vi "Argos_K_0v7.vi"(0 "PID 1 COM":refnum<visa-resource-name>="COM1", 1 "Setpoint\n START":bool, 2 "Write to File":bool, 3 "SP 1 input (°C)":dbl=20.0 min=0.0 max=1300.0, 4 "Intervall (s)":u32=1 max=600, 5 "Write/\nRead":bool=TRUE, 6 "Delay (ms)":u32=500 min=100 max=600000, 7 "Auto Tune":bool, 9 "Standby":bool, 11 "Reset\nSTOPP":bool, 12 "ON":bool=TRUE caption="OFF", 13 "Get Values":bool, 15 "File Path":path) -> (8 "(°C)":dbl format="%#.3f", 14 "SP 1 is (°C)":dbl)   [LabVIEW 2013]
doc: "1. Verwendung\n\nDas Programm dient der Steuerung und Abfrage des Thermocontrollers I3252 und dem Auslesen von zwei VC 840 Messgeräten und einem Druckmessgerät Pfeiffer Single Gauge. \nDie Messgeräte werden Standardmäßig ausgelesen und erst nach Betätigung des Schalters \"Write to File\" in einer Textdatei abgespeichert. Das Eingabefeld \"Intervall\" legt den Abstand der Messpunkte fest.\nDer Setpoint für den Thermocontroller wird erst nach Betätigung des Tasters \"Setpoint START\" übernommen und angesteuert. Er wird ind den EEPROM des Gerätes geschrieben. Die Regelung kann mit Hilfe des Schalters \"Standby\" unterbrochen werden. Durch den Taster \"Reset STOPP\" kann der Setpoint aus dem EEPROM gelöscht werden.\nDie Eingabeflächen \"Constant\" und \"Thickness\" dienen der Berechnung des spezifischen Widerstands.\nDie Eingabeflächen \"User\" und \"Sample\" werden in den Header der Textdatei übernommen.\nDer Indikator \"File Path\" zeigt den aktuellen Speicherort der Textdatei an. Dieser wird nach ausschalten des Schalters \"Write to File\" gelöscht. Bei erneuten Schreiben muss ein neuer Speicherort gewählt werden. Bei Wahl desselben Speicherorts werden sämtliche bereits gespeicherte Daten gelöscht.\n\n\n2. Erläuterungen zum Blockdiagramm\n2.1 äußere Sequenz\nDie äußerte Sequenz besteht aus fünf Frames. Der erste dient der Initialisierung der Ports. Der zweite dient als Verzögerung um dem Programm genug Zeit zu geben die Ports zu öffnen. Jedoch senden die beiden VC 840 bereits Informationen an den Computer die in einem Puffer zwischengespeichert werden. Im dritten Frame wird dieser Puffer geleert. Somit kommt es zu keinem Framing Error. Desweiteren wird in diesem Frame die Startzeit der Messungen genommen. Im vierten Frame wird die eigentliche Messung und Verarbeitung der Daten durchgeführt. Die while-Schleife wird nur durch Auftreten eines Fehlers oder durch Betätigung des Stopbuttons auf dem Front Panel in der oberen linken Ecke unterbrochen. Im fünften und letzten Frame werden die Ports wieder geschlossen und beim Auftreten eines Fehlers wird das Programm automatisch gestoppt. Falls kein Fehler auftritt wird die Sequenz von vorne abgearbeitet.\n\n2.2 while-Schleife und innere Sequenz\n2.2.1 \"Event Structure\"\n2.2.1.1 Allgemein\nDer erste Frame beinhaltet ein \"Event Structure\". Dieser reagiert auf insgesamt elf verschiedene Ereignisse. Falls keines dieser Ereignisse auftreten sollte, warte die Struktur eine Millisekunde bevor die \"Event Structure\" verlassen wird. Die übrigen Ereignisse treten ein, wenn der entsprechende Kontroller eine Werteänderung erfährt.\n\n2.2.1.2 Event: Setpoint\nDieser Case besteht von außen nach innen aus einer Stacked Sequence, einer for-Loop und einer Flat Sequence die wiederum zwei \"Case Structures\" enthält. Als erstes wird bei dem Schalter \"Setpoint START\" der Blinkmodus aktiviert und bei dem Schalter \"Read Temperature\" deaktiviert. Danach folgt das eigentliche setzen des Temperatursollwerts. In der ersten Iteration wird dem Controller I3252 ein Schreibbefehl gesendet. Theoretisch kann der Setpoint in den RAM oder in den EEPROM geschrieben werden. Diese Auswahl erfolgt mit Hilfe des Schalters \"RAM\". Da das Schreiben in den RAM -Speicher aber aus diversen Gründen nicht erwünscht ist, wurde es nicht implementiert. Eine nachträgliche Implementierung ist aber leicht möglich, in dem die untere String-Konstante \"*P012\" durch \"*W012\" ersetzt wird. An diesem Befehl wird eine fünfstellige Hexadezimalzahl angehängt, die den Sollwert wiedergibt. Der Sollwert wird vorher mit zehn multipliziert, da das Komma standardmäßig nach der ersten Ziffer festgesetzt wurde (Bsp.: 800 wird gesendet um 80 einzustellen). Dieser Befehlsstrang wird an das Gerät mittels des SubVIs \"Comm_Interface\", auf welches später noch näher eingegangen wird, weitergegeben. Der durch das Gerät zurückgegebene String wird nicht verarbeitet.\nDie zweite Iteration dient dem Auslesen des eingestellten Sollwertes. Wahlweise kann der RAM- oder der EEPROM-Speicher ausgelesen werden. Die eigentliche Verarbeitung des Ausgabestrings erfolgt durch das SubVI \"Edit Setpoint\".\nDie Implementierung zur Einstellung des zweiten Setpoints erfolgt durch kopieren der ersten beiden Fälle und ersetzen der \"1\" im Befehf durch eine \"2\" (Bsp.: \"*P012\" zu \"*P022\"). Es darf aber nicht vergessen werden, dass dann ebenfalls die Anzahl der Iterationen angepasst werden muss.\nAls letztes wird der Blinkmodus des Schalters \"Setpoint START\" wieder deaktiviert.\n\n2.2.1.3 Event: Standby\nDieses Ereignis aktiviert bzw. deaktiviert als erstes den Blinckmodus des entsprechenden Schalters und sendet danach den Befehl zum aktivieren (\"*D03\") oder zum deaktivieren (\"*E03\") des Standbymodus an den Thermocontroller.\n\n2.2.1.4 Event: Set Command \nDer in das Feld \"Command shall be\" eingegebene Befehl wird an den Thermocontroller übermittlet. Die korrekte Form des Befehls ist im \"Communication Manuel\" nachzuschlagen. Das \"*\"-Zeichen wurde allerdings schon implementiert und muss somit nicht mit eingegeben werden.\n\n2.2.1.5 Event: Reset\nIn der ersten Iteration wird der Reset-Befehl an den Thermocontroller gesendet. In Folge wird der gesamte EEPROM-Speicher gelöscht. Deshalb wird in der zweiten Iteration der Setpoint aktualisiert. Dieser Befehl hat keinen Einfluss auf den RAM-Speicher. Die anschließende Wartezeit ist auf vier Sekunden festgesetzt und wurde empirisch ermittelt. Diese Zeit benötigt das Gerät um den Reset durchzuführen und für die Kommunikation wieder zur Verfügung zu stehen.\n\n2.2.1.6 Event: Auto Tune\nEs ist festgeschrieben, dass der Setpoint für die \"Auto Tune\"-Funktion wenigstens 20°C über der aktuellen Temperatur liegt. Deshalb wird zunächst der aktuelle Temperaturwert ausgelesen. Im zweiten Schritt werden zu diesem Wert zwanzig addiert und der Setpoint wird in den RAM-Speicher geschrieben. Das Schreiben in diesen Speicher ist nötig, da die \"Auto Tune\"-Funktion\" erst nach einem Reset startet. Im dritten Schritt wird der eigentliche Befehl für den \"Auto Tune\" gesendet (siehe dazu \"Communication Manuel\" S.27). Als vierte und letzte Iteration der for-Schleife folgt der bereits erwähnte Reset-Befehl. Der Temperatursollwert, der im RAM-Speicher eingetragen ist, muss zum Schluss wieder auf 0°C gesetzt werden. Die Zeit für die Ausführung des \"Auto Tune\"-Befehls wurde empirisch ermittelt und 45 s festgesetzt.\n\n2.2.1.7 Event: Write LOW/HI\nDieses Ereignis setzt die am Analogausgang anliegende Spannung fest. Normalerweise beträgt dieser Spannungswert 0-10 V. Das angeschlossene Netzteil verträgt aber maximal nur 2,3 V. Aus diesem Grund wird der \"%HIGH\" auf 23 gesetzt. Somit beträgt die maximal anliegende Spannung nur noch 23% von der maximal möglichen, d.h 2,3V. Ein niedrigerer Wert ist jederzeit möglich, genauso wie ein höherer für den Parameter \"%LOW\". Diese werden zunächst nacheinander in den RAM-Speicher geschrieben und anschließend wieder ausgelesen.\n\n2.2.1.8 Event: Set PID\nDie Werte für den PID-Regler können sowohl mit Hilfe der \"Auto Tune\"-Funktion, als auch manuell eingestellt werden. Es wird wiederum zwischen dem Schreiben in den RAM- und dem EEPROM-Speicher unterschieden. Zunächst werden die Werte für \"P\", \"I\" und \"D\", in dieser Reihenfolge, gesetzt und danach die aktuellen Werte ausgelesen.\n\n2.2.1.9 Event: Get Values\nDieses Ereignis hat zur Folge, dass die Werte für \"P\", \"I\", \"D\", \"%LOW\", \"%HIGH\" und des Setpoints wahlweise aus dem RAM- oder EEPROM-Speicher gelesen werden. Die aktuellen Werte werden nicht nur in die entsprechenden Anzeigefelder übernommen, sondern auch in die entsprechenden Eingabefelder, mit Ausnahme des Temperatursollwerts. \n\n2.2.1.10 Event: RAM\nPrinzipiell kann zwischen dem Schreiben in den RAM- oder EEPROM-Speicher des Thermocontrollers gewählt werden. Die entsprechende Schalterposition auf dem Frontpanel zeigt den aktuell verwendeten Speicher an. Die Anzeigewerte werden bei jedem Umschalten aktualisiert und sind im entsprechenden Speicher eingetragen. Die Implementierung ist identisch mit der des Ereignisses \"Get Values\". Es gilt zu beachten, dass die Werte für \"%LOW\" und \"%HIGH\" nur in den RAM-Speicher geschrieben werden können und somit auch nur aus diesem ausgelesen werden können.\n\n2.2.1.11 Event: Set Gauge to Zero\nMit Hilfe der SubVIs \"Get Pressure\" und \"Offset Display\" werden die Werte für den alten und den neuen Offset und der durch den zweiten Drucksensor ermittelt Druck ermittelt. \n\n2.2.1.12 Event: Write to File\nSollte der Schalter \"Write to File\" aktiviert werden, d.h. Schalterposition oben, so wird zunächst durch das SubVI \"Header\" ein Header für die unter \"File Path\" definierte Datei angelegt. Alle Werte, die bereits in der entsprechenden Datei stehen, werden dabei gelöscht.\n\n2.2.2 \"Timed Structures\"\nIm dritten Frame der inneren Sequenz werden die Werte für Zeitpunkt, Temperatur, Spannung, Strom und Druck ermittelt. Damit die Werte zum gleichen Zeitpunkt aufgenommen werden, werden \"Timed Sequences\" eingesetzt. Mit dem entsprechenden Schalter auf dem Front Panel unter dem Tab \"Settings\" kann gewählt werden, ob das entsprechende Gerät ausgelesen werden soll oder nicht. Die einzelnen Sequenzen werden parallel abgearbeitet, womit die Prozesszeit von diesem Frame durch der zeitintensivsten Sequenz abhängt. Dies ist in aller Regel das Auslesen der Temperatur, da ein \"Delay\" von 500 ms oder größer benötigt wird, um den Controller ordentlich ansprechen zu können.\nDie Systemzeit wird durch das SubVI \"System Time in Seconds\" in Sekunden umgerechnet und der in dem Parameter \"Starttime\" gespeicherte Wert wird abgezogen. Somit werden die Sekunden seit dem Start des Programms gezählt.\n\n2.2.3 restlichen Frames\nIm zweiten Frame wird das Intervall zwischen den einzelnen Messwerten festgelegt. Dabei wird der Wert des Parameters \"Delay\" abgezogen. Dieser Wert beträgt im Normalfall 500 ms und ist somit nicht vernachlääsigbar.\nDer Vierte Frame beinhaltet die Umrechnung des Temperatur-Strings in einen Temperaturwert durch das SubVI \"Edit Tmperature\", die Berechnung des spezifischen Widerstands durch das SubVI \"Resistivity Calculation\" und die Überprüfung des Druckwerts. Auch werden die neu gewonnen Werte in das entsprechende Shift-Register übernommen. Falls der Druckwert einen in dem Parameter \"Pressure Limit (mbar)\" festgelegten Grenzwert überschreiten sollte, wird der Thermocontroller automatisch in den Standby-Modus versetzt. Des Weiteren wird der Schalter \"Standby\" solange gesperrt, wie der Druck oberhalb des Grenzwertes liegt. Wenn der Druck wieder unter den Grenzwert gesunken ist, wird der Standby-Befehl nicht automatisch aufgehoben, sondern muss vom Benutzer durch Betätigung des entsprechenden Schalters gegeben werden.\nIm fünften Frame werden die Diagramme erstellt. Dabei wird jedes Mal von neuem das gesamte Shift-Register als Graph dargestellt. Weiterhin werden die Messwerte in ein 1D-Array geschrieben.\nDer sechste und letzte Frame beinhaltet den eigentlich Schreibvorgang der Messwerte in eine Textdatei und die Überprüfung ob ein Fehler vorliegt.\n\n2.3 SubVIs\n2.3.1 Allgemein\nDie SubVIs für die Messgeräte VC840 und das Druckmessgerät wurden aus anderen Quellen übernommen. \n\n2.3.2 \"Header\"\nIn den Header wird zunächst das aktuelle Datum und die aktuelle Zeit übernommen. Die ausgewählte Datei wird dabei überschrieben. Danach wird der Name des Benutzers und der Probe übernommen. Zum Schluss werden die Einheiten in einer Reihe, durch einen Tabulator getrennt, in den Header geschrieben.\n\n2.3.3 \"I3252 Comm Interface\"\nDieses VI stellt die Kommunikation mit dem Thermocontroller her und gibt den Ausgabe-String zurück.\n\n2.3.4 \"I3252 Edit Setpoint\"\nIm Ausgabe-String vom Thermocontroller ist an der vierten Stelle die Stelle des Dezimalpunktes verschlüsselt. Dieses Hexadezimalzahl wird herausgefiltert und an ein \"ENUM Controller\" übergeben. Dieser weist der Hexadezimalzahl eine Nummer zu, mit welcher ein Wert aus einem Array entnommen wird. Dieser Wert dient als Quotient. Der tatsächliche Wert kann somit errechnet werden.\n\n2.3.5 \"I3252 Edit Temperature\"\nDer Temperatur-String, der vom Thermocontroller zurückgegeben wird, wird in eine Dezimalzahl umgewandelt. Manchmal kommt es aus zu Dropouts, die durch dieses Programm herausgefiltert werden. Der letzte Wert wird dabei in einer \"Feedback Node\" gehalten unter der Annahme, dass sich der Temperaturwert nicht sprunghaft ändert.\n\n2.3.6 \"Resistivity Calculation\"\nDer spezifische Widerstand wird nach folgender Formel ausgerechnet. Dabei entspricht t der Dicke der Probe und C ist eine Konstante.\nrho=C*pi*t*U/(ln( 2)*I)\n\n2.3.7 \"System Time in Seconds\"\nZunächst wird die aktuelle Systemzeit ausgelesen. Danach wird diese in Stunden, Minuten und Sekunden aufgeteilt, alles in Sekunden umgerechnet und letztendlich addiert."
uses:
  <vilib>/Platform/TimedLoop/XDataNode/timing_clust.ctl
  <vilib>/Platform/TimedLoop/XDataNode/nitl_modes.ctl
  <vilib>/Platform/TimedLoop/XDataNode/wakeup.ctl
  <vilib>/Instr/_visa.llb/VISA Configure Serial Port (Instr).vi
  <vilib>/Platform/TimedLoop/scheduler/LVUserAPI/_suppVIs/Create_1kHz_TSource.vi
  <vilib>/Utility/file.llb/Write To Spreadsheet File (DBL).vi
  <vilib>/Platform/TimedLoop/XDataNode/XDataNode.xnode
  <vilib>/Platform/TimedLoop/XDataNode/XDNodeRunTimeDep.lvlib
  Dependencies/Pfeiffer TPG261+262 Single+Dual Gauge/Dual Gauge.lvlib
panel:
  out "(°C) 2":dbl format="%#.3f"
  in  "File Path 2":path
  out "appended array":dbl[](array[numeric])
  in  "Tab Control":T1(tab)
  out "Pirani (VVP1 Scroll)":cluster{dbl[], dbl[]}(graph)
  in  "Thickness (nm)":dbl min=0.0
  in  "4PP constant":dbl min=0.0 max=5.0
  in  "Sample":string
  in  "User":string
  out "Thermocouple (Sample holder 1)":cluster{dbl[], dbl[]}(graph)
  out "current time (s)":dbl
  out "data logger intervall (s)":dbl
  out "loop time (s)":dbl
  in  "stop":bool
  out "CMR275 Baratron":cluster{dbl[], dbl[]}(graph)
  out "Pressure Baratron 2":dbl format="%#_4e"
  out "PKR251 FullRange":cluster{dbl[], dbl[]}(graph)
  out "Pressure FullRange 2":dbl format="%#_3e"
  out "Pressure Pirani 2":dbl format="%#_3e"
  out "Pressure OpenPort":cluster{dbl[], dbl[]}(graph)
  out "Pressure OpenPort2":dbl caption="current"
  in  "PID 2 COM":refnum<visa-resource-name>="COM1"
  in  "Baud Rate 2":u32=9600
  in  "Data Bits 2":u16=7 min=5 max=8 step=1
  in  "Parity 2":u16(ring)=1 items=["None", "Odd", "Even", "Mark", "Space"]
  in  "Stop Bits 2":u16(ring)=10 items=["1.0"=10, "1.5"=15, "2.0"=20]
  in  "Flow Control 2":u16(ring) items=["None"=0, "XON/XOFF"=1, "RTS/CTS"=2, "DTR/DSR"=4]
  in  "Delay (ms) 2":u32=500 min=100 max=600000
  in  "Write/\nRead 2":bool=TRUE
  out "status 2":bool caption="Status"
  out "code 2":i32 caption="Code"
  out "code":i32 caption="Code"
  out "status":bool caption="Status"
  in  "Set Gauge to Zero":bool
  out "Status Gauge 1#2":i32(ring) items=["data OK", "underrange", "overrange", "sensor error", "sensor off", "no sensor", "ID error"]
  out "Pressure Gauge 1#2":dbl format="%.3e"
  out "Pressure Gauge 1#1":dbl format="%.3e"
  out "Status Gauge 1#1":i32(ring) items=["data OK", "underrange", "overrange", "sensor error", "sensor off", "no sensor", "ID error"]
  in  "TPG 1 COM":refnum<visa-resource-name>="COM5"
  in  "Pressure Limit (mbar)":dbl=1.0 min=0.0 max=1100.0
  out "Current Offset (mbar)":dbl
  in  "ON (TPG 2)":bool=TRUE caption="OFF"
  in  "ON (TPG 1)":bool=TRUE caption="OFF"
  in  "ON":bool caption="OFF"
  in  "VC 840 2":refnum<visa-resource-name>="COM7"
  out "Reading 2":dbl format="%_4f"
  out "Mode 2":enum16{"?", "Diode", "Beep", "DC", "AC"}(ring)
  out "Unit 2":string
  in  "VC 840 1":refnum<visa-resource-name>="COM7"
  out "Reading 1":dbl format="%_4f"
  out "Mode 1":enum16{"?", "Diode", "Beep", "DC", "AC"}(ring)
  out "Unit 1":string
  out "Status 1":T2
  out "Status 2":T2
  in  "ON":bool caption="OFF"
  out "% HIGH Istwert":u32
  out "% LOW Istwert":u32
  in  "% High Sollwert":u32=23 max=24
  in  "% LOW Sollwert":u32 max=25
  in  "RAM":bool=TRUE caption="EEPROM"
  out "D (Rate) IstWert":u32
  out "I ( Reset1) Istwert":u32
  out "P (PB1) Istwert":u32 caption="actual value"
  in  "D (Rate) Sollwert":u32 max=3999
  in  "I ( Reset1) Sollwert":u32 max=3999
  in  "P (PB1) Sollwert":u32 caption="set value" max=9999
  in  "Set Command":bool
  in  "Set PID":bool
  in  "Write LOW/HI":bool
  in  "Flow Control":u16(ring) items=["None"=0, "XON/XOFF"=1, "RTS/CTS"=2, "DTR/DSR"=4]
  in  "Stop Bits":u16(ring)=10 items=["1.0"=10, "1.5"=15, "2.0"=20]
  in  "Parity":u16(ring)=1 items=["None", "Odd", "Even", "Mark", "Space"]
  in  "Data Bits":u16=7 min=5 max=8 step=1
  in  "Baud Rate":u32=9600
  out "Command output":string
  in  "Command input":string
  in  "TPG 2 COM":refnum<visa-resource-name>="COM6"
  out "Pressure Gauge 2#2":dbl format="%.3e"
  out "Pressure Gauge 2#1":dbl format="%.3e"
  out "Status Gauge 2#2":i32(ring) items=["data OK", "underrange", "overrange", "sensor error", "sensor off", "no sensor", "ID error"]
  out "Status Gauge 2#1":i32(ring) items=["data OK", "underrange", "overrange", "sensor error", "sensor off", "no sensor", "ID error"]
  out "Current":cluster{dbl[], dbl[]}(graph)
  out "Voltage":cluster{dbl[], dbl[]}(graph)
  out "Voltage (V)":dbl format="%.4e"
  out "Current (A)":dbl format="%.4e"
  out "Resistivity":cluster{dbl[], dbl[]}(graph)
  out "Resistivity (Ohm*cm)":dbl format="%.3e"
  # "set \nvalue"
  # "actual \nvalue"
  # "T (°C)"
  # "mbar"
  # "mbar"
  # "mbar"
  # "mbar"
  # "Pressure Measurement \n(Pfeiffer TPG261)"
  # "PID Controller (Omega Newport i3252)"
  # "PID Controller (Omega Newport i3252)"
  # "limit (mbar)"
  # "Multimeter\n#1 (VC 840)"
  # "Multimeter\n#2 (VC 840)"
  # "P"
  # "I"
  # "D"
  # "% Low"
  # "% High"
  # "Authors:  Daniel Schuster (sir-dan@web.de)\n                 Steffen Cornelius (s.cornelius@hzdr.de)\n                 Nico Spahn (x)\n\n                 premade SubVIs for readout of Pfeiffer gauge and VC840 Multimeters were used\n                 SubVI \"I3252_Comm_Interface\" is based on a modified Labview example\n\nRelease:  v1.0    \n\nVersion History:\n\nv1.1  -    28.06.2011\n             - Format des Files geändert von %.3f auf %g\n             - maximale Eingabewerte für PID begrenzt\nv1.2  -    12.07.2011\n             - Anzeige p,rho, U, V auf Scientific geändert\n             - y-Achse p,rho auf Log geändert\n             - numerische Zeitanzeige hinzugefügt\n             - 4PP Constant: pi/ln(2)=4,532 set as the default value\nv1.3  -    25.07.2011\n             - Zeitvariable auf EXT geändert, um Sprünge in Diagrammen loszuwerden\nv1.4  -   27.07.2011\n             - ALLE Variablen auf DBL zurückgesetzt wegen Formatierungsproblem im File\n             - Zeitberechnung neu gemacht (Tick count differenzen) -> Zeitsprünge korrigiert ?\n             - Delay/Intervall überarbeitet\nv1.5  -   05.12.2012\n                - Austausch der alten Pfeifer SubvIs durch neue -> nun alle 4 Kanäle des DualGauge\n                                                                                                         Controllers gleichzeitig auslesbar\n                - neue Pfeiffer SubVIs verwendet in Druckwertauslesung und Offset Berechnung des Baratron\n                  Druckes (COM5 Sensor1)\n                - Neuarragement des GUI -> FullRange und Baratron neben Temperatur auf Haupseite zu sehen\n                                                                   Pirani und OpenPort auf Meas.2 zu sehen\n                                                                   Diagnose Seite umfasst nun auch Widerstandsdiagramm\n                - Änderungen der Settingseite -> nun alle 4 Drucksensoren mit aktuellem Messwert und Gerätestatus\n                                                                           zu sehen\n                - The readout of the PID-Temperature Controller and the VC840 Multimeters was not modified\nv1.73  -  18.10.2013\n                - Layout Änderungen\nv.1.8   -  19.01.2014\n                - Änderung Layout Settings Tab\n                - Trennung der beiden TPG Dual Gauge Controls\n                -"
  # "Version 1.73    - last change 18.10.2013"
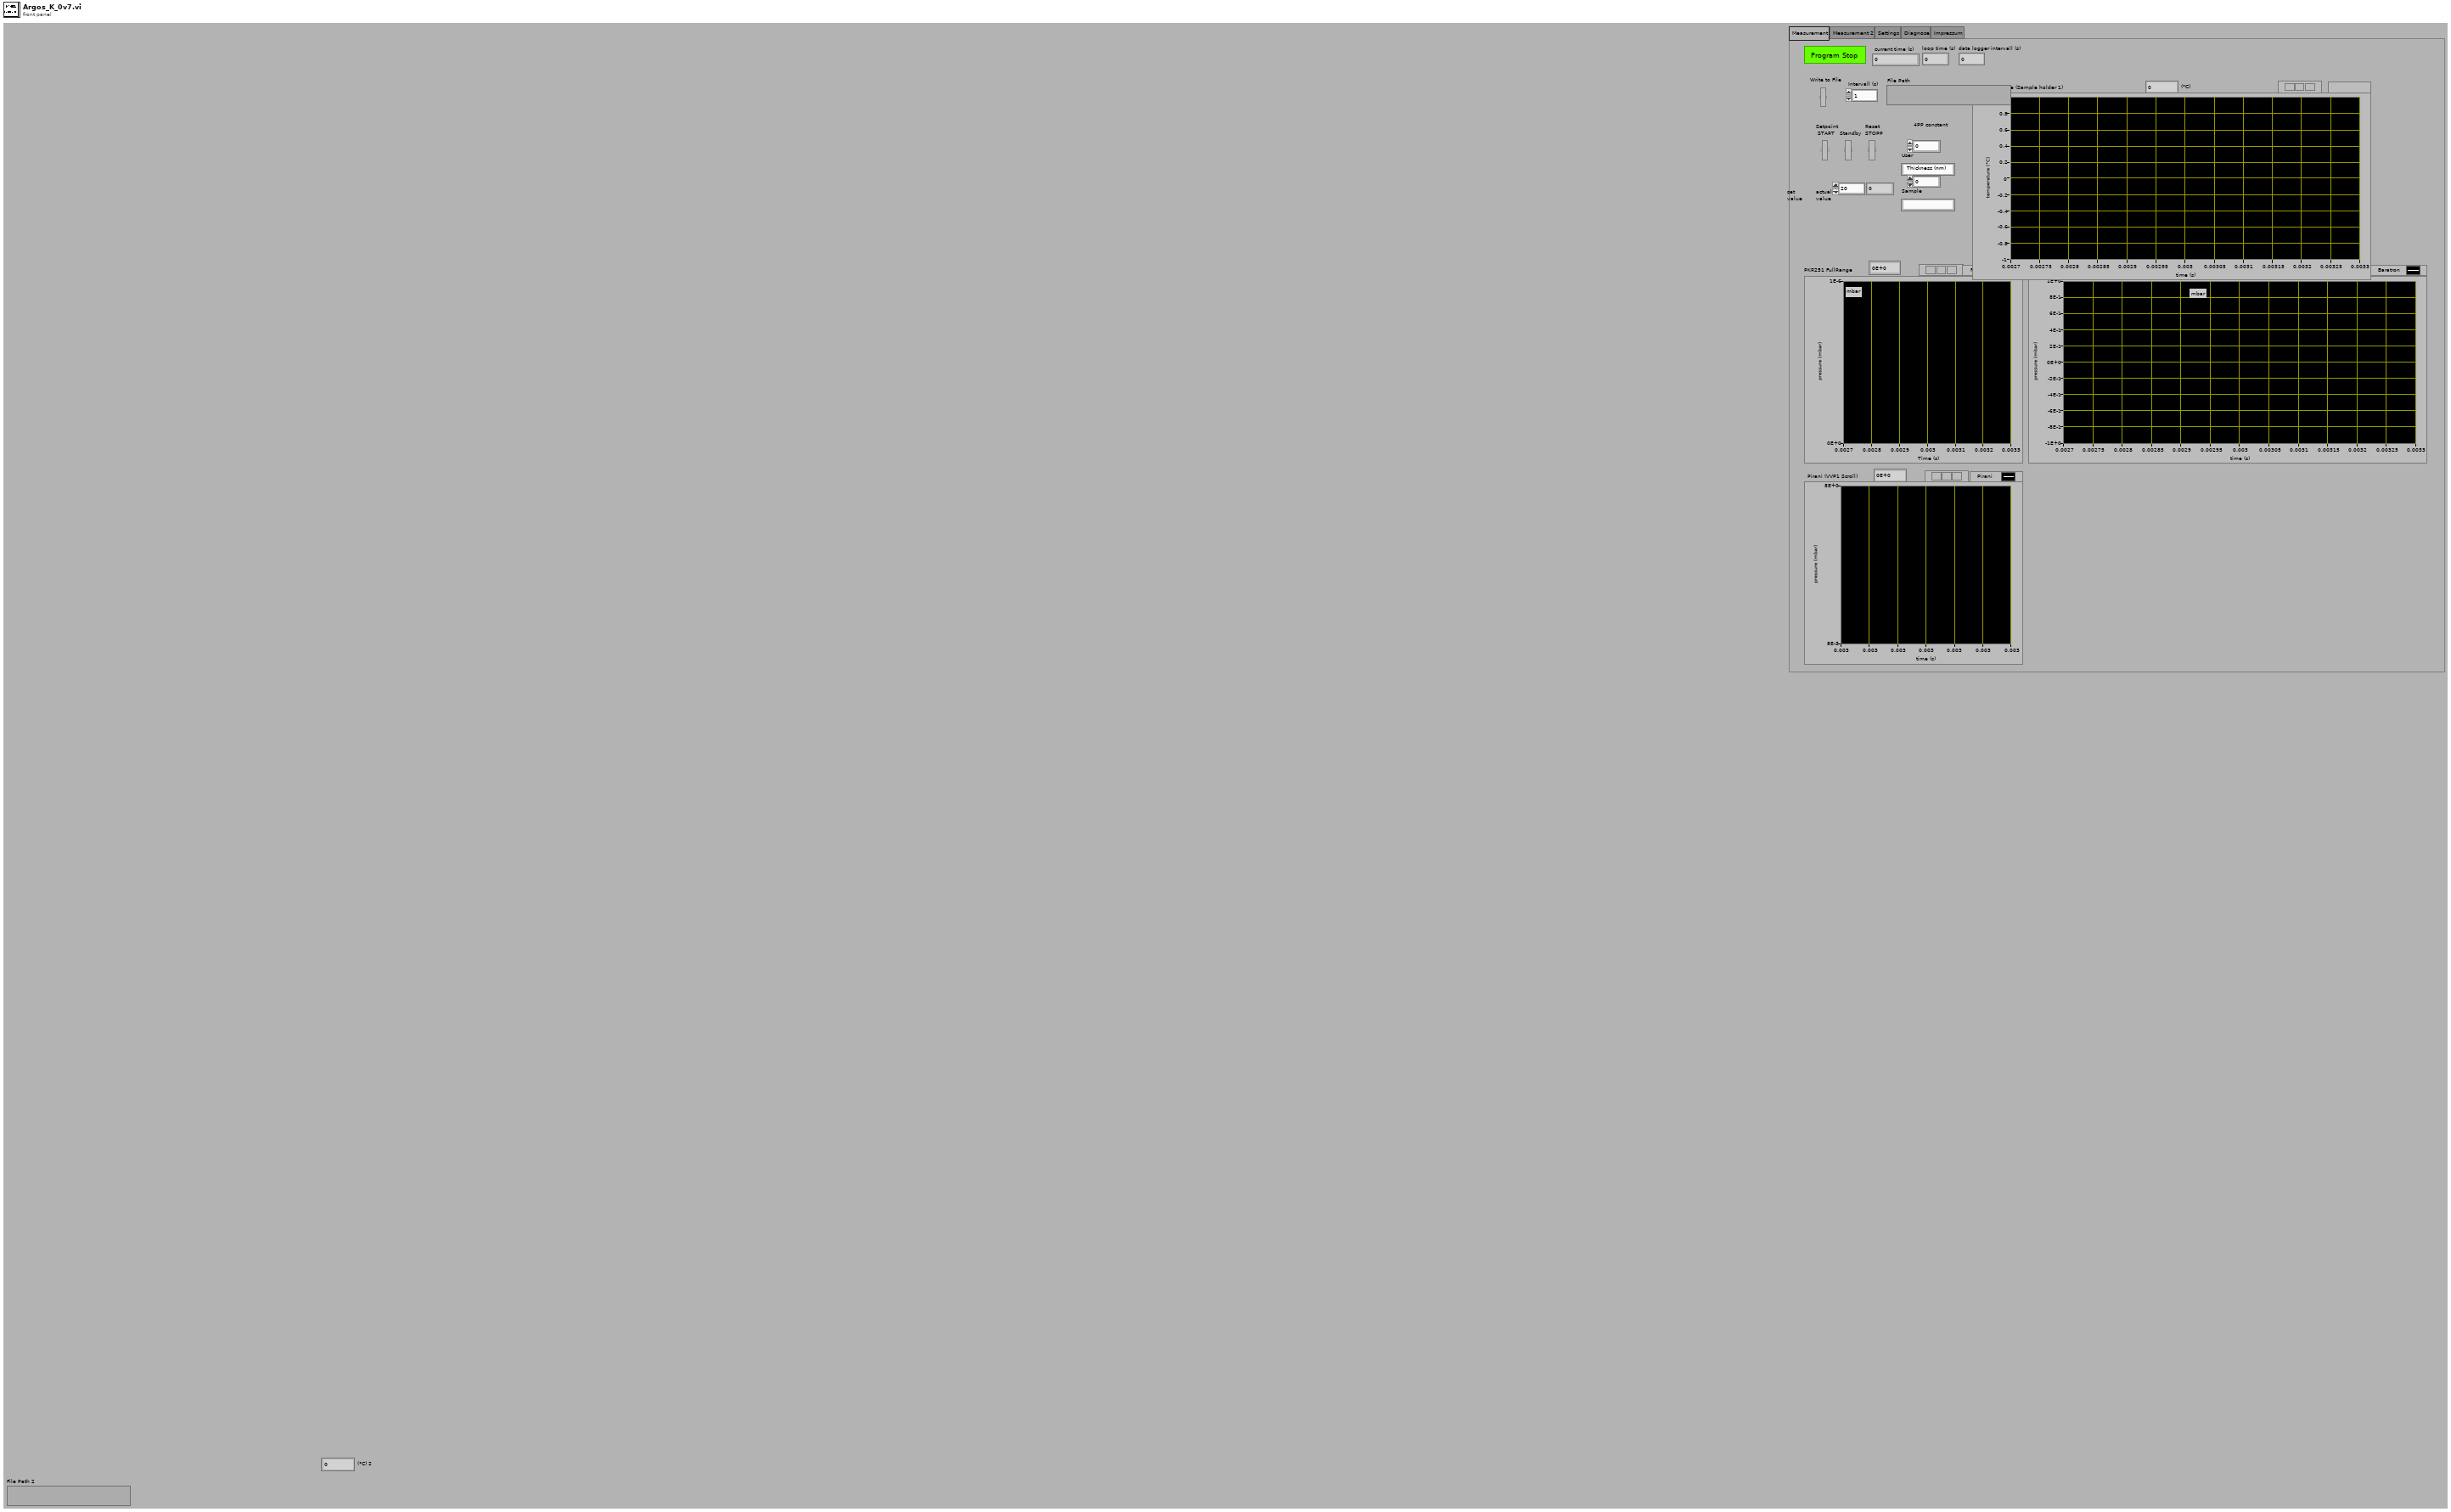
[diagram p1: front panel]
types:
  T1 = enum32{"Measurement", "Measurement 2", "Settings", "Diagnose", "Impressum"}
  T2 = cluster{"Low Bat":bool, "Auto":bool, "Delta":bool, "Hold":bool, "RS232":bool}
  T3 = typedef "XDNodeRunTimeDep.lvlib/timing_clust.ctl" = cluster{"Expected End [f-1]":u64, "Actual End [f-1]":u64, "Finished Late? [f-1]":bool, "Expected End [i-1]":u64, "Actual End [i-1]":u64, "Finished Late? [i-1]":bool, "Expected Start [i]":u64, "Actual Start [i]":u64, "Expected Start [f]":u64, "Actual Start [f]":u64, "Source Name":string, "Structure Name":string, "Period":i64, "Deadline":i64, "Offset":i64, "Start":i64, "Priority":i32, "Timeout":i32, "Mode":T4, "Wakeup Reason":T5, "Error":errorcluster, "Source Type":string, "Secondary Source Type":string, "Global End Time":u64, "Global Start Time":u64, "Frame Duration":u64, "Iteration Duration":u64, "Assigned CPU":i32, "I/O Scan Engine Mode":u32}
  T4 = typedef "XDNodeRunTimeDep.lvlib/nitl_modes.ctl" = enum32{"No Change", "Process missed periods, maintain original phase", "Discard missed periods, maintain original phase", "Process missed periods, ignore original phase", "Discard missed periods, ignore original phase"}
  T5 = typedef "XDNodeRunTimeDep.lvlib/wakeup.ctl" = enum32{"Normal", "Aborted", "Asynchronous wakeup", "Timing source error", "Timed loop error", "Timeout"}
  T6 = enum8{"Enabled", "Disabled", "Disabled and Grayed Out"}
  T7 = cluster{"VISA resource name out":refnum<visa-resource-name>, "error out":errorcluster, "Delay (ms)":u32, "Write/\nRead":bool}
  T8 = cluster{"VISA resource name out":refnum<visa-resource-name>, "error out":errorcluster, "Delay (ms) 2":u32, "Write/\nRead 2":bool}
  T9 = cluster{"TPG 2 COM":refnum<visa-resource-name>, "error out":errorcluster}
  T10 = cluster{"COM out":refnum<visa-resource-name>, "Cluster (Ausgang)":errorcluster}
  T11 = cluster{"Pressure Gauge#1":dbl, "Pressure Gauge#2":dbl}
  T12 = cluster{"TPG 1 COM":refnum<visa-resource-name>, "error out":errorcluster}
  T13 = cluster{"COM out":refnum<visa-resource-name>, "error out":errorcluster, "COM out":refnum<visa-resource-name>, "error out":errorcluster}
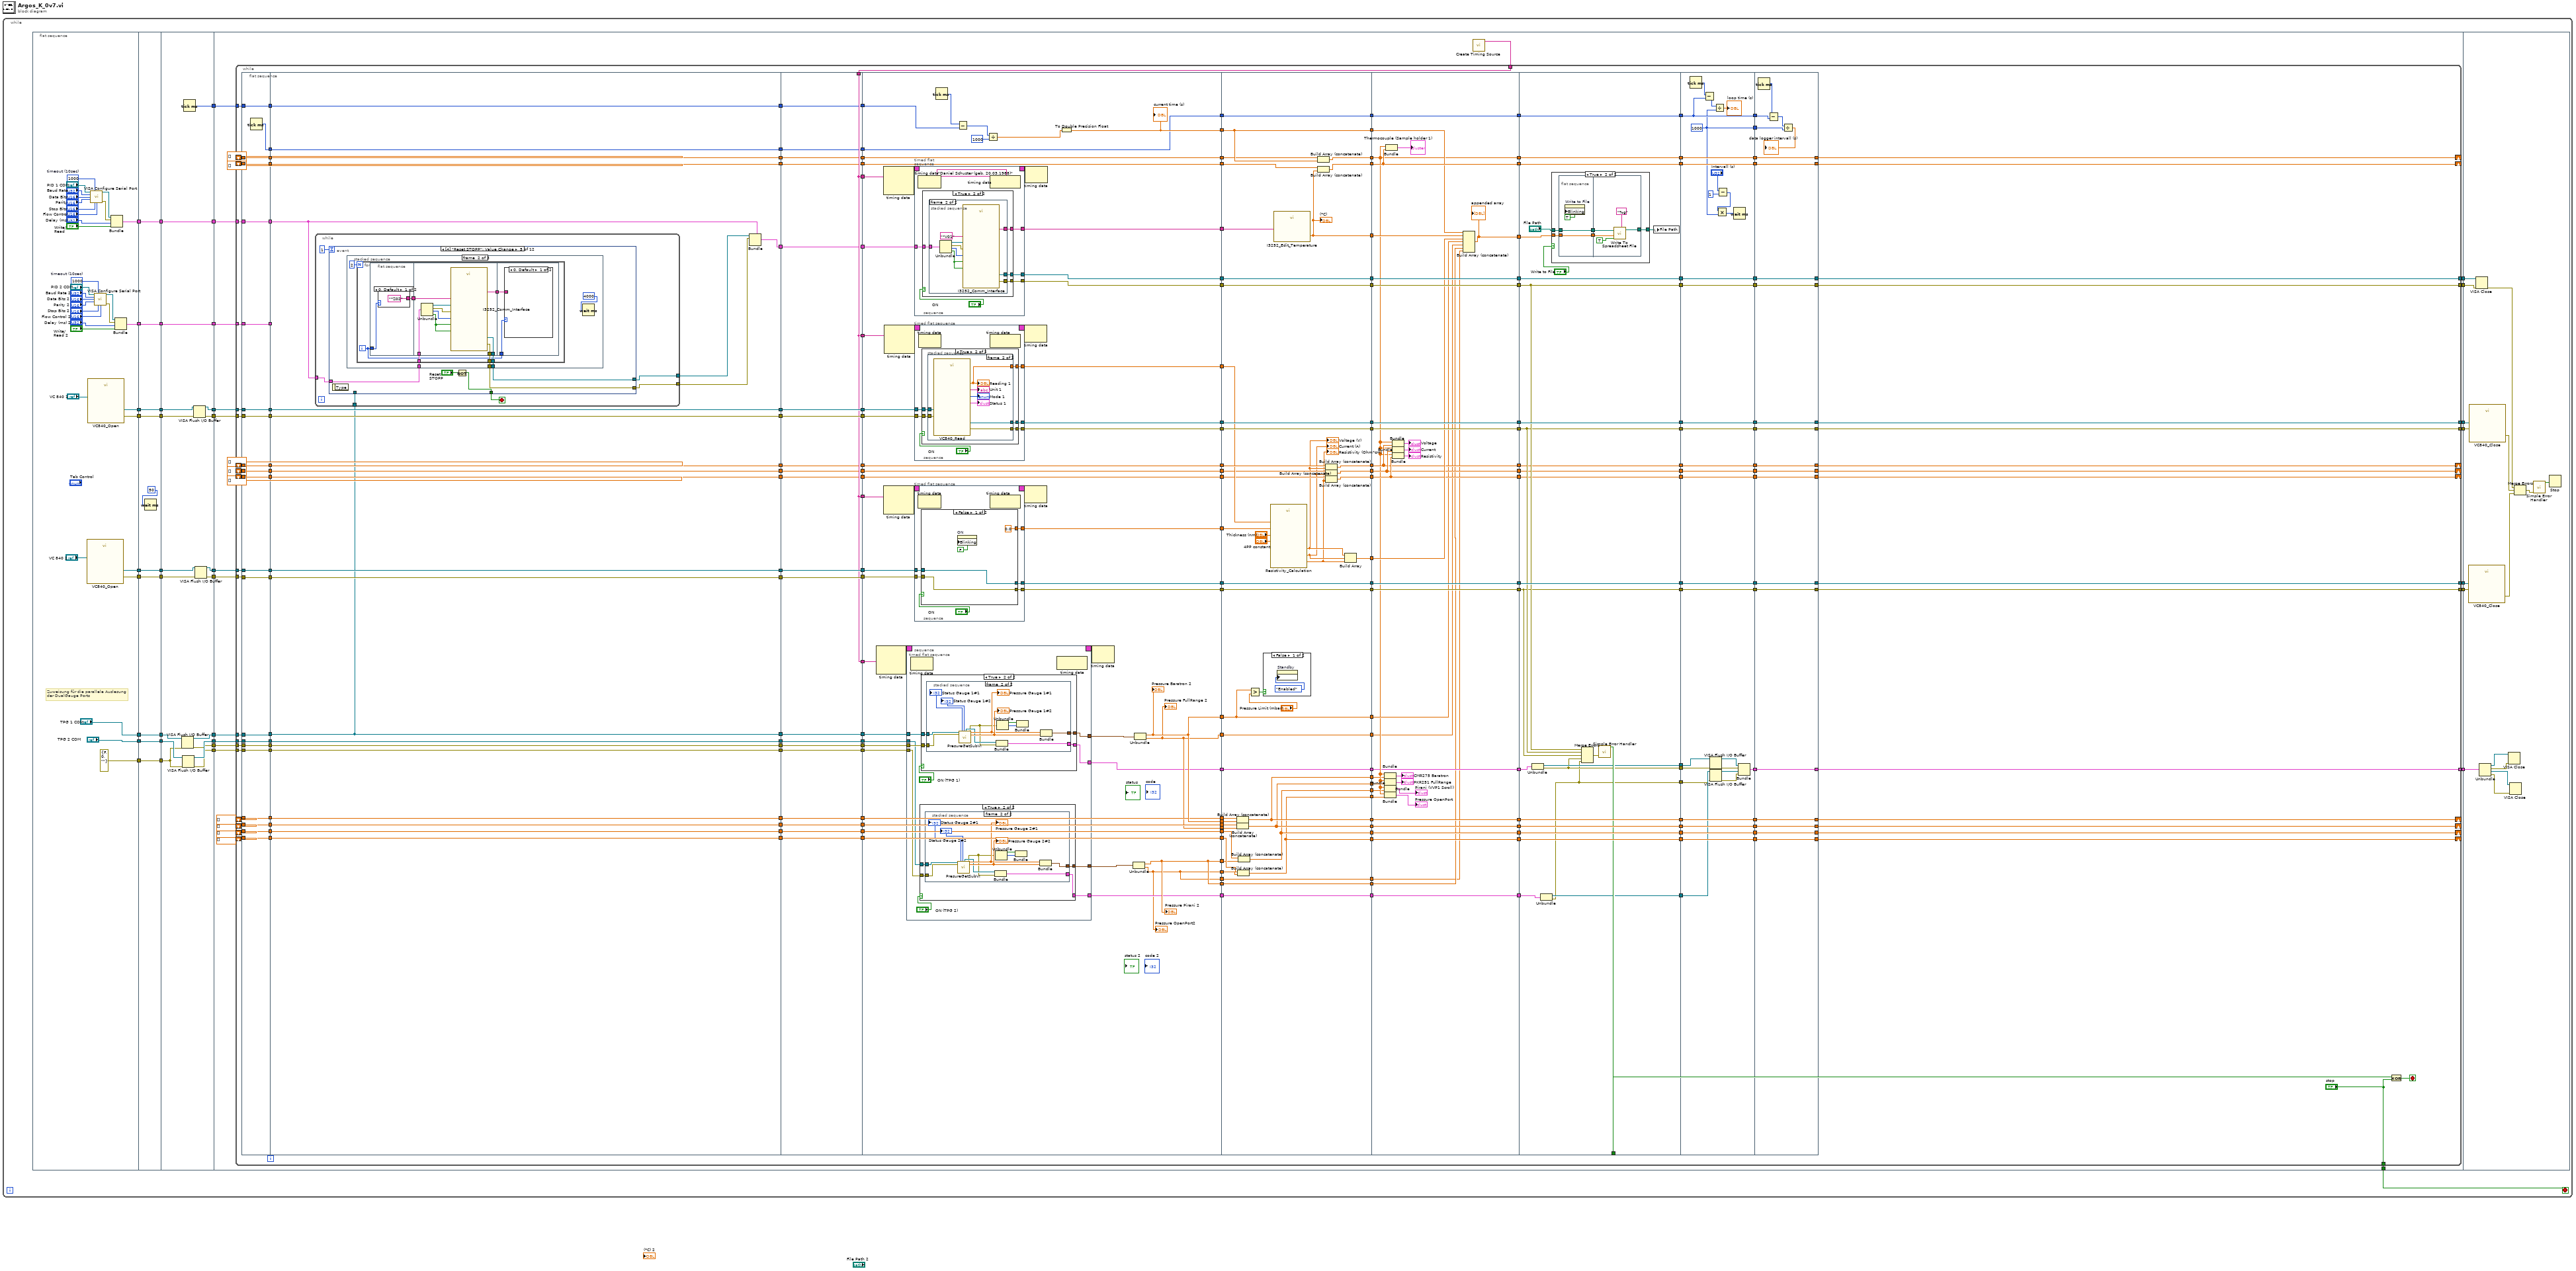
[diagram p0: block diagram]
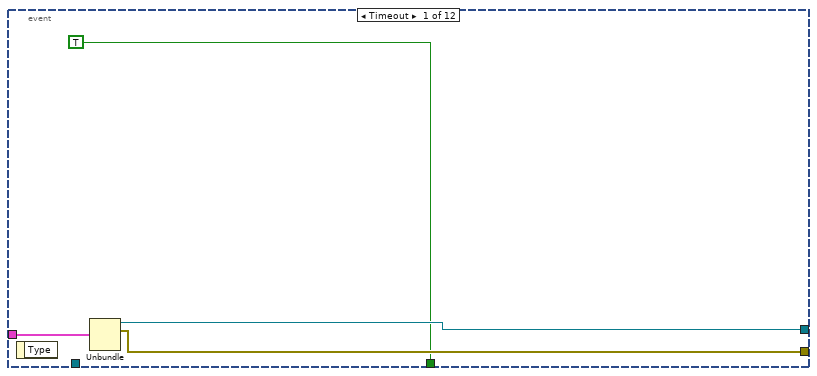
[diagram p2: hidden frame]
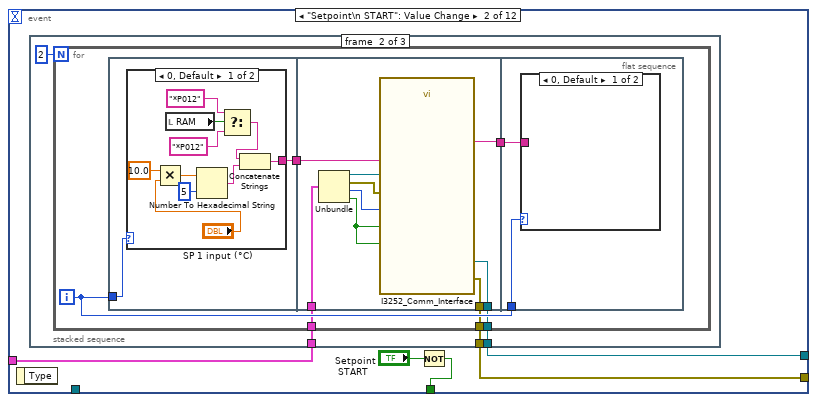
[diagram p3: hidden frame]
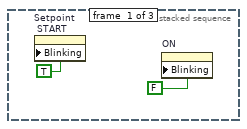
[diagram p4: hidden frame]
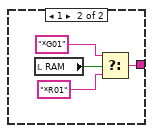
[diagram p5: hidden frame]
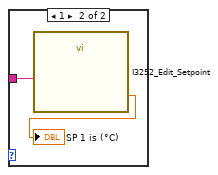
[diagram p6: hidden frame]
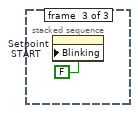
[diagram p7: hidden frame]
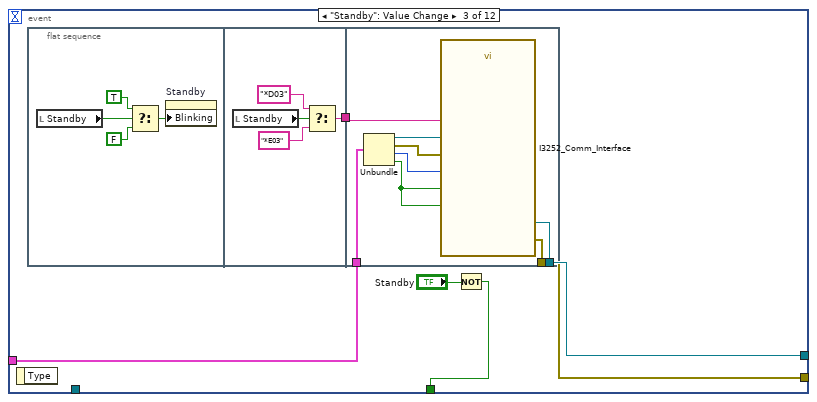
[diagram p8: hidden frame]
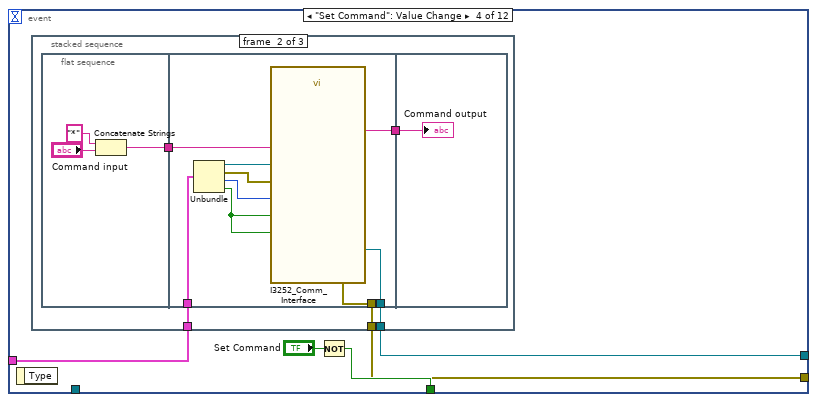
[diagram p9: hidden frame]
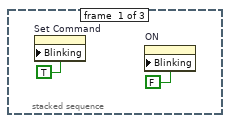
[diagram p10: hidden frame]
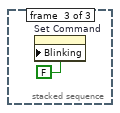
[diagram p11: hidden frame]
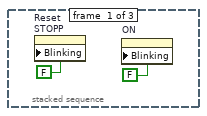
[diagram p12: hidden frame]
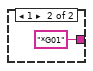
[diagram p13: hidden frame]
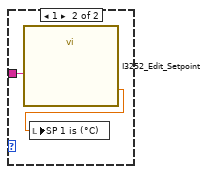
[diagram p14: hidden frame]
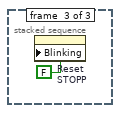
[diagram p15: hidden frame]
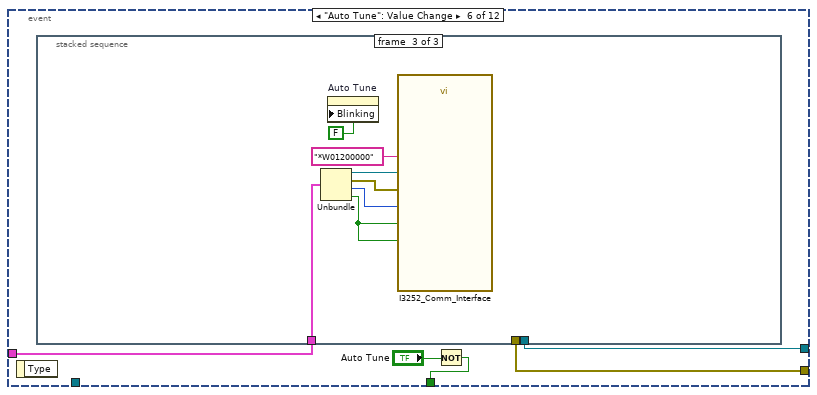
[diagram p16: hidden frame]
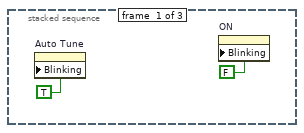
[diagram p17: hidden frame]
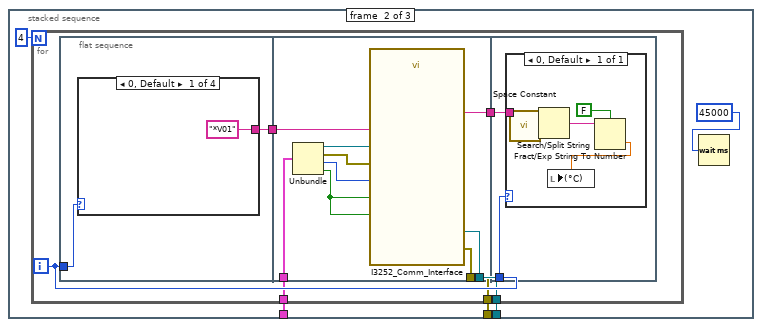
[diagram p18: hidden frame]
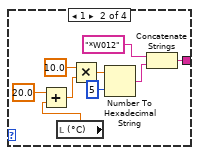
[diagram p19: hidden frame]
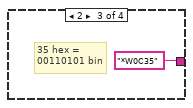
[diagram p20: hidden frame]
diagram:
  n1 = while {
    stop <- w9 stop-if-true
    n2 = flat-sequence {
      tunnel: [w69] -> w37
      tunnel: [w70] -> w36
      tunnel: [w55] -> w35
      tunnel: [w68] -> w34
      tunnel: [w67] -> w33
      tunnel: ["TPG 1 COM"] -> w32
      tunnel: ["TPG 2 COM"] -> w31
      tunnel: [errorcluster {"status"=FALSE, "code"=0, "source"=""} ("Fehler (Eingang)")] -> w6
      tunnel: [w38] -> w1
      tunnel: w37 -> [w80]
      tunnel: [w80] -> w30
      tunnel: w36 -> [w79]
      tunnel: [w79] -> w29
      tunnel: w35 -> [w78]
      tunnel: [w78] -> w28
      tunnel: w34 -> [w77]
      tunnel: [w77] -> w27
      tunnel: w33 -> [w76]
      tunnel: [w76] -> w26
      tunnel: [w74] -> w25
      tunnel: w32 -> [w74]
      tunnel: [w73] -> w24
      tunnel: w31 -> [w73]
      tunnel: [w72] -> w7
      tunnel: w6 -> [w72]
      tunnel: [w71] -> w2
      tunnel: w1 -> [w71]
      tunnel: w30 -> [w92]
      tunnel: [w91] -> w23
      tunnel: w29 -> [w93]
      tunnel: [w90] -> w22
      tunnel: w28 -> [w98]
      tunnel: [w98] -> w21
      tunnel: w27 -> [w95]
      tunnel: [w96] -> w20
      tunnel: w26 -> [w94]
      tunnel: [w97] -> w19
      tunnel: [w89] -> w18
      tunnel: [w87] -> w17
      tunnel: w25 -> [w88]
      tunnel: [w86] -> w16
      tunnel: w24 -> [w85]
      tunnel: w7 -> [w84]
      tunnel: [w83] -> w5
      tunnel: [w82] -> w4
      tunnel: [w81] -> w3
      tunnel: w2 -> [w81]
      tunnel: w23 -> [w127]
      tunnel: w22 -> [w126]
      tunnel: w21 -> [w125]
      tunnel: w20 -> [w123]
      tunnel: w19 -> [w122]
      tunnel: [w121] -> w15
      tunnel: [w120] -> w14
      tunnel: [w119] -> w13
      tunnel: [w118] -> w12
      tunnel: [w117] -> w11
      tunnel: [w116] -> w10
      tunnel: w18 -> [w110]
      tunnel: w17 -> [w109]
      tunnel: w16 -> [w108]
      tunnel: [w103] -> w9
      tunnel: [w102] -> w8
      tunnel: w5 -> [w101]
      tunnel: w4 -> [w100]
      tunnel: w3 -> [w99]
      tunnel: w15 -> [w1337]
      tunnel: w14 -> [w1336]
      tunnel: w13 -> [w1339]
      tunnel: w12 -> [w1338]
      tunnel: w11 -> [w1341]
      tunnel: w10 -> [w1340]
      tunnel: w8 -> [w1334]
      frame #0 {
        w39 = u32 1000  # timeout (10sec)
        w56 = u32 1000  # timeout (10sec)
        # "Zuweisung für die parallele Auslesung\nder DualGauge Ports"
        n3 = call "VC840_Open.vi"("VISA resource name"="VC 840 2") -> ("error out"=w67:errorcluster, "VISA resource name out"=w68:refnum<visa-resource-name>)  [unwired: 1 in, 8 out]
        n4 = call "VC840_Open.vi"("VISA resource name"="VC 840 1") -> ("error out"=w70:errorcluster, "VISA resource name out"=w69:refnum<visa-resource-name>)  [unwired: 1 in, 8 out]
        n5 = call-poly "VISA Configure Serial Port"("VISA resource name"="PID 1 COM", "timeout (10sec)"=w56, "baud rate (9600)"="Baud Rate", "data bits (8)"="Data Bits", "parity (0:none)"="Parity", "stop bits (10: 1 bit)"="Stop Bits", "flow control (0:none)"="Flow Control") -> ("VISA resource name out"=w65:refnum<visa-resource-name>, "error out"=w66:errorcluster)  [unwired: 2 in, 5 out]
        n6 = call-poly "VISA Configure Serial Port"("VISA resource name"="PID 2 COM", "timeout (10sec)"=w39, "baud rate (9600)"="Baud Rate 2", "data bits (8)"="Data Bits 2", "parity (0:none)"="Parity 2", "stop bits (10: 1 bit)"="Stop Bits 2", "flow control (0:none)"="Flow Control 2") -> ("VISA resource name out"=w48:refnum<visa-resource-name>, "error out"=w49:errorcluster)  [unwired: 2 in, 5 out]
        n7 = Bundle("VISA resource name out"=w65, "error out"=w66, "Delay (ms)"="Delay (ms)", "Write/\nRead"="Write/\nRead") -> (w55:T7)  [unwired: 1 in]
        n8 = Bundle("VISA resource name out"=w48, "error out"=w49, "Delay (ms) 2"="Delay (ms) 2", "Write/\nRead 2"="Write/\nRead 2") -> (w38:T8)  [unwired: 1 in]
      }
      frame #1 {
        n9 = Wait (ms)(milliseconds to wait=u32 50) -> ()  [unwired: 1 out]
      }
      frame #2 {
        n10 = VISA Flush I/O Buffer(VISA resource name=w88, error in (no error)=w84) -> (VISA resource name out=w87:refnum<visa-resource-name>, error out=w83:errorcluster)  [unwired: 1 in]
        n11 = VISA Flush I/O Buffer(VISA resource name=w85, error in (no error)=w84) -> (VISA resource name out=w86:refnum<visa-resource-name>, error out=w82:errorcluster)  [unwired: 1 in]
        n12 = Tick Count (ms)() -> (millisecond timer value=w89:u32)
        n13 = VISA Flush I/O Buffer(VISA resource name=w92, error in (no error)=w93) -> (VISA resource name out=w91:refnum<visa-resource-name>, error out=w90:errorcluster)  [unwired: 1 in]
        n14 = VISA Flush I/O Buffer(VISA resource name=w95, error in (no error)=w94) -> (VISA resource name out=w96:refnum<visa-resource-name>, error out=w97:errorcluster)  [unwired: 1 in]
      }
      frame #3 {
        n15 = call-poly <vilib>:"Create Timing Source.vi"() -> ("name (out)"=w124:string)  [unwired: 10 in, 1 out]
        n16 = while {
          tunnel: w127 -> [w348]
          tunnel: w126 -> [w347]
          tunnel: w125 -> [w346]
          tunnel: w124 -> [w339]
          tunnel: w123 -> [w332]
          tunnel: w122 -> [w331]
          tunnel: [w327] -> w121
          tunnel: [w326] -> w120
          tunnel: [w324] -> w119
          tunnel: [w322] -> w118
          tunnel: [w320] -> w117
          tunnel: [w318] -> w116
          shift-right: [w291] -> _
          shift-left: dbl[] [] -> [w296]
          shift-right: [w269] -> _
          shift-left: dbl[] [] -> [w304]
          shift-right: [w293] -> _
          shift-left: dbl[] [] -> [w300]
          shift-right: [w266] -> _
          shift-left: dbl[] [] -> [w303]
          shift-right: [w263] -> _
          shift-left: dbl[] [] -> [w302]
          tunnel: w110 -> [w257]
          tunnel: w109 -> [w213]
          tunnel: w108 -> [w209]
          shift-right: [w167] -> _
          shift-left: dbl[] [] -> [w197]
          shift-right: [w165] -> _
          shift-left: dbl[] [] -> [w195]
          shift-right: [w163] -> _
          shift-left: dbl[] [] -> [w193]
          shift-right: [w161] -> _
          shift-left: dbl[] [] -> [w191]
          tunnel: ["stop"] -> w103
          tunnel: [w155] -> w102
          tunnel: w101 -> [w150]
          tunnel: w100 -> [w148]
          tunnel: w99 -> [w128]
          stop <- w154 stop-if-true
          n17 = flat-sequence {
            tunnel: w257 -> [w359]
            tunnel: w296 -> [w360]
            tunnel: w300 -> [w361]
            tunnel: w302 -> [w362]
            tunnel: w303 -> [w363]
            tunnel: w304 -> [w364]
            tunnel: w331 -> [w365]
            tunnel: w332 -> [w366]
            tunnel: w346 -> [w367]
            tunnel: w347 -> [w368]
            tunnel: w348 -> [w369]
            tunnel: [w369] -> w256
            tunnel: [w368] -> w255
            tunnel: [w367] -> w254
            tunnel: [w366] -> w253
            tunnel: [w365] -> w252
            tunnel: [w364] -> w251
            tunnel: [w363] -> w250
            tunnel: [w362] -> w249
            tunnel: [w361] -> w248
            tunnel: [w360] -> w247
            tunnel: [w359] -> w246
            tunnel: [w358] -> w228
            tunnel: [w357] -> w214
            tunnel: w213 -> [w357]
            tunnel: [w356] -> w210
            tunnel: w209 -> [w356]
            tunnel: [w355] -> w198
            tunnel: w197 -> [w355]
            tunnel: [w354] -> w196
            tunnel: w195 -> [w354]
            tunnel: [w353] -> w194
            tunnel: w193 -> [w353]
            tunnel: [w352] -> w192
            tunnel: w191 -> [w352]
            tunnel: [w351] -> w151
            tunnel: w150 -> [w351]
            tunnel: [w350] -> w149
            tunnel: w148 -> [w350]
            tunnel: [w349] -> w129
            tunnel: w128 -> [w349]
            tunnel: [w392] -> w345
            tunnel: [w391] -> w343
            tunnel: [w387] -> w341
            tunnel: [w386] -> w336
            tunnel: [w385] -> w334
            tunnel: [w384] -> w301
            tunnel: [w383] -> w297
            tunnel: [w382] -> w277
            tunnel: [w381] -> w274
            tunnel: [w380] -> w272
            tunnel: [w379] -> w258
            tunnel: w256 -> [w392]
            tunnel: w255 -> [w391]
            tunnel: w254 -> [w390]
            tunnel: w253 -> [w386]
            tunnel: w252 -> [w385]
            tunnel: w251 -> [w382]
            tunnel: w250 -> [w381]
            tunnel: w249 -> [w380]
            tunnel: w248 -> [w384]
            tunnel: w247 -> [w383]
            tunnel: w246 -> [w379]
            tunnel: [w378] -> w229
            tunnel: w228 -> [w378]
            tunnel: w214 -> [w376]
            tunnel: [w376] -> w211
            tunnel: w210 -> [w377]
            tunnel: [w377] -> w207
            tunnel: w198 -> [w375]
            tunnel: w196 -> [w374]
            tunnel: w194 -> [w373]
            tunnel: w192 -> [w372]
            tunnel: [w375] -> w190
            tunnel: [w374] -> w186
            tunnel: [w373] -> w183
            tunnel: [w372] -> w182
            tunnel: w151 -> [w371]
            tunnel: w149 -> [w370]
            tunnel: [w371] -> w146
            tunnel: [w370] -> w144
            tunnel: w129 -> [_]
            tunnel: w345 -> [w917]
            tunnel: [w917] -> w344
            tunnel: w343 -> [w916]
            tunnel: [w916] -> w342
            tunnel: w341 -> [w912]
            tunnel: [w912] -> w340
            tunnel: w339 -> [w913]
            tunnel: [w913] -> w338
            tunnel: [w913] -> w337
            tunnel: w336 -> [w915]
            tunnel: [w915] -> w335
            tunnel: w334 -> [w914]
            tunnel: [w914] -> w333
            tunnel: [w913] -> w330
            tunnel: [w913] -> w316
            tunnel: w301 -> [w911]
            tunnel: [w911] -> w299
            tunnel: w297 -> [w910]
            tunnel: [w910] -> w294
            tunnel: [w909] -> w278
            tunnel: w277 -> [w909]
            tunnel: [w908] -> w275
            tunnel: w274 -> [w908]
            tunnel: [w907] -> w273
            tunnel: w272 -> [w907]
            tunnel: [w906] -> w259
            tunnel: w258 -> [w906]
            tunnel: [w905] -> w230
            tunnel: w229 -> [w905]
            tunnel: [w904] -> w212
            tunnel: w211 -> [w904]
            tunnel: [w903] -> w208
            tunnel: w207 -> [w903]
            tunnel: w190 -> [w902]
            tunnel: [w902] -> w189
            tunnel: [w901] -> w187
            tunnel: w186 -> [w901]
            tunnel: [w900] -> w185
            tunnel: w183 -> [w900]
            tunnel: w182 -> [w899]
            tunnel: [w899] -> w181
            tunnel: [w898] -> w147
            tunnel: w146 -> [w898]
            tunnel: [w897] -> w145
            tunnel: w144 -> [w897]
            tunnel: [w940] -> w315
            tunnel: w344 -> [w969]
            tunnel: w342 -> [w968]
            tunnel: w340 -> [w965]
            tunnel: w338 -> [w964]
            tunnel: w337 -> [w963]
            tunnel: w335 -> [w953]
            tunnel: w333 -> [w952]
            tunnel: w330 -> [w954]
            tunnel: [w950] -> w314
            tunnel: [w951] -> w313
            tunnel: [w962] -> w312
            tunnel: [w961] -> w311
            tunnel: [w960] -> w310
            tunnel: [w959] -> w309
            tunnel: w316 -> [w949]
            tunnel: [w948] -> w308
            tunnel: [w947] -> w307
            tunnel: [w931] -> w306
            tunnel: [w946] -> w305
            tunnel: w299 -> [w945]
            tunnel: [w945] -> w298
            tunnel: [w944] -> w295
            tunnel: w294 -> [w944]
            tunnel: w278 -> [w943]
            tunnel: [w943] -> w276
            tunnel: w275 -> [w942]
            tunnel: w273 -> [w941]
            tunnel: [w942] -> w271
            tunnel: [w941] -> w270
            tunnel: w259 -> [w939]
            tunnel: [w935] -> w231
            tunnel: w230 -> [w935]
            tunnel: w212 -> [w933]
            tunnel: w208 -> [w932]
            tunnel: [w926] -> w206
            tunnel: [w931] -> w205
            tunnel: [w929] -> w204
            tunnel: [w927] -> w203
            tunnel: w189 -> [w930]
            tunnel: [w930] -> w188
            tunnel: w187 -> [w929]
            tunnel: w185 -> [w928]
            tunnel: [w928] -> w184
            tunnel: w181 -> [w927]
            tunnel: [w926] -> w159
            tunnel: [w925] -> w156
            tunnel: w147 -> [w924]
            tunnel: w145 -> [w923]
            tunnel: [w920] -> w140
            tunnel: [w918] -> w139
            tunnel: [w920] -> w138
            tunnel: [w919] -> w134
            tunnel: [w918] -> w131
            tunnel: w315 -> [w1179]
            tunnel: [w1176] -> w289
            tunnel: w314 -> [w1192]
            tunnel: [w1192] -> w288
            tunnel: w313 -> [w1191]
            tunnel: [w1191] -> w287
            tunnel: w312 -> [w1190]
            tunnel: [w1190] -> w286
            tunnel: w311 -> [w1189]
            tunnel: [w1189] -> w285
            tunnel: w310 -> [w1188]
            tunnel: [w1188] -> w284
            tunnel: w309 -> [w1187]
            tunnel: [w1187] -> w283
            tunnel: [w1180] -> w282
            tunnel: w308 -> [w1173]
            tunnel: w307 -> [w1181]
            tunnel: w306 -> [w1180]
            tunnel: w305 -> [w1182]
            tunnel: [w1179] -> w281
            tunnel: w298 -> [w1178]
            tunnel: w295 -> [w1177]
            tunnel: [w1175] -> w280
            tunnel: [w1163] -> w279
            tunnel: w276 -> [w1174]
            tunnel: w271 -> [w1171]
            tunnel: w270 -> [w1170]
            tunnel: [w1172] -> w267
            tunnel: [w1169] -> w264
            tunnel: [w1168] -> w261
            tunnel: [w1164] -> w260
            tunnel: [w1162] -> w232
            tunnel: w231 -> [w1162]
            tunnel: w206 -> [w1161]
            tunnel: w205 -> [w1160]
            tunnel: w204 -> [w1159]
            tunnel: w203 -> [w1157]
            tunnel: [w1155] -> w202
            tunnel: [w1154] -> w201
            tunnel: [w1153] -> w200
            tunnel: [w1152] -> w199
            tunnel: w188 -> [w1156]
            tunnel: w184 -> [w1158]
            tunnel: [w1155] -> w180
            tunnel: [w1154] -> w179
            tunnel: [w1153] -> w178
            tunnel: [w1152] -> w177
            tunnel: [w1151] -> w160
            tunnel: w159 -> [w1151]
            tunnel: [w1150] -> w157
            tunnel: w156 -> [w1150]
            tunnel: w140 -> [w1149]
            tunnel: w139 -> [w1148]
            tunnel: w138 -> [w1147]
            tunnel: [w1147] -> w137
            tunnel: [w1146] -> w135
            tunnel: w134 -> [w1146]
            tunnel: w131 -> [w1145]
            tunnel: [w1145] -> w130
            tunnel: w289 -> [w1226]
            tunnel: [w1233] -> w329
            tunnel: [w1232] -> w328
            tunnel: w288 -> [w1232]
            tunnel: [w1227] -> w325
            tunnel: w287 -> [w1227]
            tunnel: [w1231] -> w323
            tunnel: w286 -> [w1231]
            tunnel: [w1230] -> w321
            tunnel: w285 -> [w1230]
            tunnel: [w1229] -> w319
            tunnel: w284 -> [w1229]
            tunnel: [w1228] -> w317
            tunnel: w283 -> [w1228]
            tunnel: w282 -> [w1215]
            tunnel: w281 -> [w1216]
            tunnel: w280 -> [w1211]
            tunnel: [w1211] -> w292
            tunnel: w279 -> [w1217]
            tunnel: [w1217] -> w290
            tunnel: [w1219] -> w268
            tunnel: w267 -> [w1219]
            tunnel: [w1220] -> w265
            tunnel: w264 -> [w1220]
            tunnel: [w1221] -> w262
            tunnel: w261 -> [w1221]
            tunnel: w260 -> [w1225]
            tunnel: [w1214] -> w233
            tunnel: w232 -> [w1214]
            tunnel: w202 -> [w1210]
            tunnel: w201 -> [w1209]
            tunnel: w200 -> [w1208]
            tunnel: w199 -> [w1207]
            tunnel: w180 -> [w1206]
            tunnel: w179 -> [w1205]
            tunnel: w178 -> [w1204]
            tunnel: w177 -> [w1203]
            tunnel: [w1206] -> w175
            tunnel: [w1205] -> w173
            tunnel: [w1204] -> w171
            tunnel: [w1203] -> w169
            tunnel: w160 -> [w1202]
            tunnel: [w1201] -> w158
            tunnel: w157 -> [w1201]
            tunnel: w137 -> [w1198]
            tunnel: [w1197] -> w136
            tunnel: w135 -> [w1197]
            tunnel: w130 -> [w1196]
            tunnel: w329 -> [w1246]
            tunnel: w328 -> [w1261]
            tunnel: w325 -> [w1255]
            tunnel: w323 -> [w1260]
            tunnel: w321 -> [w1257]
            tunnel: w319 -> [w1259]
            tunnel: w317 -> [w1258]
            tunnel: w292 -> [w1251]
            tunnel: w290 -> [w1250]
            tunnel: w268 -> [w1249]
            tunnel: w265 -> [w1248]
            tunnel: w262 -> [w1247]
            tunnel: [w1240] -> w153
            tunnel: [w1261] -> w245
            tunnel: [w1255] -> w244
            tunnel: [w1260] -> w243
            tunnel: [w1257] -> w242
            tunnel: [w1259] -> w241
            tunnel: [w1258] -> w240
            tunnel: [w1251] -> w239
            tunnel: [w1250] -> w238
            tunnel: [w1249] -> w237
            tunnel: [w1248] -> w236
            tunnel: [w1247] -> w235
            tunnel: [w1245] -> w234
            tunnel: w233 -> [w1245]
            tunnel: [w1244] -> w176
            tunnel: w175 -> [w1244]
            tunnel: [w1243] -> w174
            tunnel: w173 -> [w1243]
            tunnel: [w1242] -> w172
            tunnel: w171 -> [w1242]
            tunnel: [w1241] -> w170
            tunnel: w169 -> [w1241]
            tunnel: w158 -> [w1239]
            tunnel: [w1238] -> w143
            tunnel: [w1237] -> w142
            tunnel: w136 -> [w1236]
            tunnel: [w1235] -> w133
            tunnel: [w1234] -> w132
            tunnel: w245 -> [w1308]
            tunnel: w244 -> [w1307]
            tunnel: w243 -> [w1306]
            tunnel: w242 -> [w1305]
            tunnel: w241 -> [w1304]
            tunnel: w240 -> [w1303]
            tunnel: w239 -> [w1302]
            tunnel: w238 -> [w1301]
            tunnel: w237 -> [w1300]
            tunnel: w236 -> [w1299]
            tunnel: w235 -> [w1298]
            tunnel: w234 -> [w1291]
            tunnel: [w1308] -> w227
            tunnel: [w1307] -> w226
            tunnel: [w1306] -> w225
            tunnel: [w1305] -> w224
            tunnel: [w1304] -> w223
            tunnel: [w1303] -> w222
            tunnel: [w1302] -> w221
            tunnel: [w1301] -> w220
            tunnel: [w1300] -> w219
            tunnel: [w1299] -> w218
            tunnel: [w1298] -> w217
            tunnel: [w1291] -> w216
            tunnel: [w1290] -> w215
            tunnel: w176 -> [w1288]
            tunnel: w174 -> [w1287]
            tunnel: w172 -> [w1286]
            tunnel: w170 -> [w1285]
            tunnel: [w1288] -> w168
            tunnel: [w1287] -> w166
            tunnel: [w1286] -> w164
            tunnel: [w1285] -> w162
            tunnel: w143 -> [w1284]
            tunnel: w142 -> [w1283]
            tunnel: [w1278] -> w141
            tunnel: w133 -> [w1277]
            tunnel: w132 -> [w1276]
            tunnel: [w1319] -> w263
            tunnel: [w1320] -> w266
            tunnel: [w1321] -> w269
            tunnel: [w1322] -> w291
            tunnel: [w1323] -> w293
            tunnel: [w1324] -> w318
            tunnel: [w1325] -> w320
            tunnel: [w1326] -> w322
            tunnel: [w1327] -> w324
            tunnel: [w1328] -> w326
            tunnel: [w1329] -> w327
            tunnel: w227 -> [w1329]
            tunnel: w226 -> [w1328]
            tunnel: w225 -> [w1327]
            tunnel: w224 -> [w1326]
            tunnel: w223 -> [w1325]
            tunnel: w222 -> [w1324]
            tunnel: w221 -> [w1323]
            tunnel: w220 -> [w1322]
            tunnel: w219 -> [w1321]
            tunnel: w218 -> [w1320]
            tunnel: w217 -> [w1319]
            tunnel: w216 -> [w1315]
            tunnel: w215 -> [w1314]
            tunnel: [w1313] -> w167
            tunnel: w168 -> [w1313]
            tunnel: [w1312] -> w165
            tunnel: w166 -> [w1312]
            tunnel: [w1311] -> w163
            tunnel: w164 -> [w1311]
            tunnel: [w1310] -> w161
            tunnel: w162 -> [w1310]
            tunnel: [w1309] -> w155
            tunnel: w141 -> [w1309]
            frame #0 {
              n18 = Tick Count (ms)() -> (millisecond timer value=w358:u32)
            }
            frame #1 {
              n19 = while {
                tunnel: w390 -> [w397]
                tunnel: [w396] -> w389
                tunnel: [w395] -> w388
                tunnel: w376 -> [w393]
                stop <- w398 stop-if-true
                n20 = event shown="[4] \"Reset STOPP\": Value Change" {
                  selector: _ -> [_ _ _ _ _ _ _ _ _ _ _ _]
                  dyn-events: _ -> [_ _ _ _ _ _ _ _ _ _ _ _]
                  timeout: 1 -> [_ _ _ _ _ _ _ _ _ _ _ _]
                  tunnel: [TRUE ("Set Gauge to Zero") w406 w455 w476 w502 w537 w593 w644 w723 w794 "Set Gauge to Zero" _] -> w398
                  tunnel: w397 -> [w402 w405 w452 w474 w498 w536 w589 w642 w721 w792 w869 w891]
                  tunnel: [w401 w404 w451 w473 w500 w534 w591 w641 w720 w791 w868 w890] -> w396
                  tunnel: [w400 w403 w450 w472 w499 w535 w590 w640 w719 w790 w867 w889] -> w395
                  tunnel: w393 -> [_ _ _ _ _ _ _ _ _ _ w865 _]
                  event Timeout {
                    n21 = event-data() -> ()  [unwired: 1 in, 1 out]
                    n22 = Unbundle(w402) -> ("VISA resource name out"=w401:refnum<visa-resource-name>, "error out"=w400:errorcluster)  [unwired: 2 out]
                  }
                  event "Setpoint\n START": Value Change {
                    n23 = event-data() -> ()  [unwired: 1 in, 1 out]
                    n24 = stacked-sequence {
                      tunnel: w405 -> [_ w412 _]
                      tunnel: [_ w411 _] -> w403
                      tunnel: [_ w410 _] -> w404
                      frame #0 {
                        n25 = property on="Setpoint\n START" class="Bool"("Blinking"=TRUE) -> ()  [unwired: 2 in, 2 out]
                        n26 = property on="ON" class="Bool (strict)"("Blinking"=FALSE) -> ()  [unwired: 2 in, 2 out]
                      }
                      frame #1 {
                        n27 = for {
                          N: 2 -> [_]
                          tunnel: w412 -> [w416]
                          tunnel: [w415] -> w411
                          tunnel: [w414] -> w410
                          i -> [w418]
                          n28 = flat-sequence {
                            tunnel: [w421] -> w417
                            tunnel: w418 -> [w420]
                            tunnel: [w439] -> w419
                            tunnel: w417 -> [w438]
                            tunnel: w416 -> [w440]
                            tunnel: [w437] -> w415
                            tunnel: [w436] -> w414
                            tunnel: w419 -> [w446]
                            tunnel: w418 -> [w445]
                            frame #0 {
                              n29 = case shown="0, Default" w420 {
                                tunnel: [w430 w432] -> w421
                                frame 0, Default {
                                n30 = Multiply(x=10.0, y="SP 1 input (°C)") -> (x*y=w427:dbl)
                                n31 = local read "RAM"() -> (w425:bool)
                                n32 = Number To Hexadecimal String(1:i16 5 ("width (-)"), 2:w427) -> (0:w429:string)
                                n33 = Select(t="*P012", s=w425, f="*P012") -> (s? t:f=w422:string)
                                n34 = Concatenate Strings(w422, w429) -> (w430:string)
                                }
                                frame 1 {
                                n35 = local read "RAM"() -> (w435:bool)
                                n36 = Select(t="*G01", s=w435, f="*R01") -> (s? t:f=w432:string)
                                }
                              }
                            }
                            frame #1 {
                              n37 = Unbundle(w440) -> ("VISA resource name out"=w441:refnum<visa-resource-name>, "error out"=w443:errorcluster, "Delay (ms)"=w442:u32, "Write/\nRead"=w444:bool)
                              n38 = call "I3252_Comm_Interface.vi"("VISA resource name in"=w441, "error in"=w443, "Delay (ms)"=w442, "Write"=w444, "String to Write"=w438, "Read"=w444) -> ("VISA resource name out"=w436:refnum<visa-resource-name>, "error out"=w437:errorcluster, "Read String"=w439:string)  [unwired: 2 in]
                            }
                            frame #2 {
                              n39 = case shown="0, Default" w445 {
                                tunnel: w446 -> [_ w448]
                                frame 0, Default {
                                }
                                frame 1 {
                                n40 = call "I3252_Edit_Setpoint.vi"("Read String"=w448) -> ("Setpoint is"=→"SP 1 is (°C)":dbl)
                                }
                              }
                            }
                          }
                        }
                      }
                      frame #2 {
                        n41 = property on="Setpoint\n START" class="Bool"("Blinking"=FALSE) -> ()  [unwired: 2 in, 2 out]
                      }
                    }
                    n42 = Not(x="Setpoint\n START") -> (.not. x?=w406:bool)
                  }
                  event "Standby": Value Change {
                    n43 = event-data() -> ()  [unwired: 1 in, 1 out]
                    n44 = flat-sequence {
                      tunnel: [w463] -> w453
                      tunnel: w453 -> [w467]
                      tunnel: w452 -> [w466]
                      tunnel: [w465] -> w450
                      tunnel: [w464] -> w451
                      frame #0 {
                        n45 = local read "Standby"() -> (w456:bool)
                        n46 = Select(t=TRUE, s=w456, f=FALSE) -> (s? t:f=w459:bool)
                        n47 = property on="Standby" class="Bool (strict)"("Blinking"=w459) -> ()  [unwired: 2 in, 2 out]
                      }
                      frame #1 {
                        n48 = local read "Standby"() -> (w461:bool)
                        n49 = Select(t="*D03", s=w461, f="*E03") -> (s? t:f=w463:string)
                      }
                      frame #2 {
                        n50 = Unbundle(w466) -> ("VISA resource name out"=w468:refnum<visa-resource-name>, "error out"=w470:errorcluster, "Delay (ms)"=w469:u32, "Write/\nRead"=w471:bool)
                        n51 = call "I3252_Comm_Interface.vi"("VISA resource name in"=w468, "error in"=w470, "Delay (ms)"=w469, "Write"=w471, "String to Write"=w467, "Read"=w471) -> ("VISA resource name out"=w464:refnum<visa-resource-name>, "error out"=w465:errorcluster)  [unwired: 2 in, 1 out]
                      }
                    }
                    n52 = Not(x="Standby") -> (.not. x?=w455:bool)
                  }
                  event "Set Command": Value Change {
                    n53 = event-data() -> ()  [unwired: 1 in, 1 out]
                    n54 = stacked-sequence {
                      tunnel: w474 -> [_ w481 _]
                      tunnel: [_ w480 _] -> w473
                      tunnel: [_ w479 _] -> w472
                      frame #0 {
                        n55 = property on="Set Command" class="Bool"("Blinking"=TRUE) -> ()  [unwired: 2 in, 2 out]
                        n56 = property on="ON" class="Bool (strict)"("Blinking"=FALSE) -> ()  [unwired: 2 in, 2 out]
                      }
                      frame #1 {
                        n57 = flat-sequence {
                          tunnel: [w486] -> w483
                          tunnel: [w489] -> w482
                          tunnel: w483 -> [w490]
                          tunnel: w481 -> [w491]
                          tunnel: [w488] -> w480
                          tunnel: [w487] -> _
                          tunnel: [w487] -> w479
                          tunnel: w482 -> [w496]
                          frame #0 {
                            n58 = Concatenate Strings("*", "Command input") -> (w486:string)
                          }
                          frame #1 {
                            n59 = Unbundle(w491) -> ("VISA resource name out"=w495:refnum<visa-resource-name>, "error out"=w493:errorcluster, "Delay (ms)"=w494:u32, "Write/\nRead"=w492:bool)
                            n60 = call "I3252_Comm_Interface.vi"("VISA resource name in"=w495, "error in"=w493, "Delay (ms)"=w494, "Write"=w492, "String to Write"=w490, "Read"=w492) -> ("VISA resource name out"=w488:refnum<visa-resource-name>, "error out"=w487:errorcluster, "Read String"=w489:string)  [unwired: 2 in]
                          }
                          frame #2 {
                            "Command output" <- w496
                          }
                        }
                      }
                      frame #2 {
                        n61 = property on="Set Command" class="Bool"("Blinking"=FALSE) -> ()  [unwired: 2 in, 2 out]
                      }
                    }
                    n62 = Not(x="Set Command") -> (.not. x?=w476:bool)
                  }
                  event "Reset\nSTOPP": Value Change {
                    n63 = event-data() -> ()  [unwired: 1 in, 1 out]
                    n64 = stacked-sequence {
                      tunnel: [_ w509 _] -> w499
                      tunnel: [_ w508 _] -> w500
                      tunnel: w498 -> [_ w506 _]
                      frame #0 {
                        n65 = property on="Reset\nSTOPP" class="Bool"("Blinking"=FALSE) -> ()  [unwired: 2 in, 2 out]
                        n66 = property on="ON" class="Bool (strict)"("Blinking"=FALSE) -> ()  [unwired: 2 in, 2 out]
                      }
                      frame #1 {
                        n67 = for {
                          N: 2 -> [_]
                          tunnel: [w515] -> w509
                          tunnel: [w514] -> w508
                          tunnel: w506 -> [w513]
                          i -> [w511]
                          n68 = flat-sequence {
                            tunnel: w511 -> [w517]
                            tunnel: [w516] -> w512
                            tunnel: [w522] -> w515
                            tunnel: [w523] -> w514
                            tunnel: w513 -> [w524]
                            tunnel: w512 -> [w521]
                            tunnel: [w520] -> w510
                            tunnel: w511 -> [w530]
                            tunnel: w510 -> [w529]
                            frame #0 {
                              n69 = case shown="0, Default" w517 {
                                tunnel: ["*Z02" "*G01"] -> w516
                                frame 0, Default {
                                }
                                frame 1 {
                                }
                              }
                            }
                            frame #1 {
                              n70 = Unbundle(w524) -> ("VISA resource name out"=w525:refnum<visa-resource-name>, "error out"=w527:errorcluster, "Delay (ms)"=w526:u32, "Write/\nRead"=w528:bool)
                              n71 = call "I3252_Comm_Interface.vi"("VISA resource name in"=w525, "error in"=w527, "Delay (ms)"=w526, "Write"=w528, "String to Write"=w521, "Read"=w528) -> ("VISA resource name out"=w523:refnum<visa-resource-name>, "error out"=w522:errorcluster, "Read String"=w520:string)  [unwired: 2 in]
                            }
                            frame #2 {
                              n72 = case shown="0, Default" w530 {
                                tunnel: w529 -> [_ w532]
                                frame 0, Default {
                                }
                                frame 1 {
                                n73 = call "I3252_Edit_Setpoint.vi"("Read String"=w532) -> ("Setpoint is"=w531:dbl)
                                n74 = local write "SP 1 is (°C)"(w531) -> ()
                                }
                              }
                            }
                          }
                        }
                        n75 = Wait (ms)(milliseconds to wait=u32 4000) -> ()  [unwired: 1 out]
                      }
                      frame #2 {
                        n76 = property on="Reset\nSTOPP" class="Bool"("Blinking"=FALSE) -> ()  [unwired: 2 in, 2 out]
                      }
                    }
                    n77 = Not(x="Reset\nSTOPP") -> (.not. x?=w502:bool)
                  }
                  event "Auto Tune": Value Change {
                    n78 = event-data() -> ()  [unwired: 1 in, 1 out]
                    n79 = stacked-sequence {
                      tunnel: w536 -> [_ w543 w588]
                      tunnel: [_ w542 _] -> w535
                      tunnel: [_ w541 _] -> w534
                      frame #0 {
                        n80 = property on="Auto Tune" class="Bool"("Blinking"=TRUE) -> ()  [unwired: 2 in, 2 out]
                        n81 = property on="ON" class="Bool (strict)"("Blinking"=FALSE) -> ()  [unwired: 2 in, 2 out]
                      }
                      frame #1 {
                        n82 = for {
                          N: 4 -> [_]
                          tunnel: [w548] -> w541
                          tunnel: [w547] -> w542
                          tunnel: w543 -> [w546]
                          i -> [w551]
                          n83 = flat-sequence {
                            tunnel: w551 -> [w553]
                            tunnel: [w552] -> w549
                            tunnel: w549 -> [w568]
                            tunnel: [w567] -> w550
                            tunnel: [w570] -> w548
                            tunnel: [w569] -> w547
                            tunnel: w546 -> [w566]
                            tunnel: w551 -> [w576]
                            tunnel: w550 -> [w575]
                            frame #0 {
                              n84 = case shown="0, Default" w553 {
                                tunnel: ["*V01" w556 "*W0C35" "*Z02"] -> w552
                                frame 0, Default {
                                }
                                frame 1 {
                                n85 = local read "(°C)"() -> (w555:dbl)
                                n86 = Add(x=20.0, y=w555) -> (x+y=w562:dbl)
                                n87 = Multiply(x=10.0, y=w562) -> (x*y=w559:dbl)
                                n88 = Number To Hexadecimal String(1:i16 5 ("width (-)"), 2:w559) -> (0:w558:string)
                                n89 = Concatenate Strings("*W012", w558) -> (w556:string)
                                }
                                frame 2 {
                                # "35 hex = \n00110101 bin"
                                }
                                frame 3 {
                                }
                              }
                            }
                            frame #1 {
                              n90 = Unbundle(w566) -> ("VISA resource name out"=w574:refnum<visa-resource-name>, "error out"=w572:errorcluster, "Delay (ms)"=w573:u32, "Write/\nRead"=w571:bool)
                              n91 = call "I3252_Comm_Interface.vi"("VISA resource name in"=w574, "error in"=w572, "Delay (ms)"=w573, "Write"=w571, "String to Write"=w568, "Read"=w571) -> ("VISA resource name out"=w570:refnum<visa-resource-name>, "error out"=w569:errorcluster, "Read String"=w567:string)  [unwired: 2 in]
                            }
                            frame #2 {
                              n92 = case shown="0, Default" w576 {
                                tunnel: w575 -> [w578]
                                frame 0, Default {
                                n93 = call <vilib>:"Space Constant.vi"() -> ("String"=w581:string)
                                n94 = Search/Split String(string=w578, search string/char (-)=w581) -> (match + rest of string=w580:string)  [unwired: 1 in, 2 out]
                                n95 = Fract/Exp String To Number(use system decimal point (T)=FALSE, string=w580) -> (number=w577:dbl)  [unwired: 2 in, 1 out]
                                n96 = local write "(°C)"(w577) -> ()
                                }
                              }
                            }
                          }
                        }
                        n97 = Wait (ms)(milliseconds to wait=u32 45000) -> ()  [unwired: 1 out]
                      }
                      frame #2 {
                        n98 = Unbundle(w588) -> ("VISA resource name out"=w587:refnum<visa-resource-name>, "error out"=w585:errorcluster, "Delay (ms)"=w586:u32, "Write/\nRead"=w584:bool)
                        n99 = property on="Auto Tune" class="Bool"("Blinking"=FALSE) -> ()  [unwired: 2 in, 2 out]
                        n100 = call "I3252_Comm_Interface.vi"("VISA resource name in"=w587, "error in"=w585, "Delay (ms)"=w586, "Write"=w584, "String to Write"="*W01200000", "Read"=w584) -> ()  [unwired: 2 in, 3 out]
                      }
                    }
                    n101 = Not(x="Auto Tune") -> (.not. x?=w537:bool)
                  }
                  event "Write LOW/HI": Value Change {
                    n102 = event-data() -> ()  [unwired: 1 in, 1 out]
                    n103 = stacked-sequence {
                      tunnel: [_ w598 _] -> w591
                      tunnel: [_ w597 _] -> w590
                      tunnel: w589 -> [_ w596 _]
                      frame #0 {
                        n104 = property on="Write LOW/HI" class="Bool"("Blinking"=TRUE) -> ()  [unwired: 2 in, 2 out]
                        n105 = property on="ON" class="Bool (strict)"("Blinking"=FALSE) -> ()  [unwired: 2 in, 2 out]
                      }
                      frame #1 {
                        n106 = for {
                          N: 4 -> [_]
                          tunnel: [w602] -> w598
                          tunnel: [w601] -> w597
                          tunnel: w596 -> [w600]
                          i -> [w604]
                          n107 = flat-sequence {
                            tunnel: w604 -> [w606]
                            tunnel: [w607] -> w603
                            tunnel: w603 -> [w621]
                            tunnel: [w622] -> w605
                            tunnel: [w624] -> w602
                            tunnel: [w623] -> w601
                            tunnel: w600 -> [w620]
                            tunnel: w605 -> [w630]
                            tunnel: w604 -> [w629]
                            frame #0 {
                              n108 = case shown="1" w606 {
                                tunnel: [w609 w615 "*R27" "*R28"] -> w607
                                frame 0, Default {
                                n109 = Number To Hexadecimal String(1:i16 2 ("width (-)"), 2:"% LOW Sollwert") -> (0:w610:string)
                                n110 = Concatenate Strings("*W27", w610) -> (w609:string)
                                }
                                frame 1 {
                                n111 = Number To Hexadecimal String(1:i16 2 ("width (-)"), 2:"% High Sollwert") -> (0:w616:string)
                                n112 = Concatenate Strings("*W28", w616) -> (w615:string)
                                }
                                frame 2 {
                                }
                                frame 3 {
                                }
                              }
                            }
                            frame #1 {
                              n113 = Unbundle(w620) -> ("VISA resource name out"=w628:refnum<visa-resource-name>, "error out"=w626:errorcluster, "Delay (ms)"=w627:u32, "Write/\nRead"=w625:bool)
                              n114 = call "I3252_Comm_Interface.vi"("VISA resource name in"=w628, "error in"=w626, "Delay (ms)"=w627, "Write"=w625, "String to Write"=w621, "Read"=w625) -> ("VISA resource name out"=w624:refnum<visa-resource-name>, "error out"=w623:errorcluster, "Read String"=w622:string)  [unwired: 2 in]
                            }
                            frame #2 {
                              n115 = case shown="0, Default" w629 {
                                tunnel: w630 -> [_ w634 w638]
                                frame 0, Default {
                                }
                                frame 2 {
                                n116 = String Subset(string=w634, offset (0)=3) -> (substring=w632:string)  [unwired: 1 in]
                                n117 = Hexadecimal String To Number(string=w632) -> (number=→"% LOW Istwert":u32)  [unwired: 2 in, 1 out]
                                }
                                frame 3 {
                                n118 = String Subset(string=w638, offset (0)=3) -> (substring=w636:string)  [unwired: 1 in]
                                n119 = Hexadecimal String To Number(string=w636) -> (number=→"% HIGH Istwert":u32)  [unwired: 2 in, 1 out]
                                }
                              }
                            }
                          }
                        }
                      }
                      frame #2 {
                        n120 = property on="Write LOW/HI" class="Bool"("Blinking"=FALSE) -> ()  [unwired: 2 in, 2 out]
                      }
                    }
                    n121 = Not(x="Write LOW/HI") -> (.not. x?=w593:bool)
                  }
                  event "Set PID": Value Change {
                    n122 = event-data() -> ()  [unwired: 1 in, 1 out]
                    n123 = stacked-sequence {
                      tunnel: w642 -> [_ w649 _]
                      tunnel: [_ w648 _] -> w641
                      tunnel: [_ w647 _] -> w640
                      frame #0 {
                        n124 = property on="Set PID" class="Bool"("Blinking"=TRUE) -> ()  [unwired: 2 in, 2 out]
                        n125 = property on="ON" class="Bool (strict)"("Blinking"=FALSE) -> ()  [unwired: 2 in, 2 out]
                      }
                      frame #1 {
                        n126 = for {
                          N: 6 -> [_]
                          tunnel: w649 -> [w653]
                          tunnel: [w652] -> w648
                          tunnel: [w651] -> w647
                          i -> [w655]
                          n127 = flat-sequence {
                            tunnel: w655 -> [w657]
                            tunnel: [w658] -> w654
                            tunnel: w654 -> [w699]
                            tunnel: [w695] -> w656
                            tunnel: w653 -> [w698]
                            tunnel: [w697] -> w651
                            tunnel: [w696] -> w652
                            tunnel: w656 -> [w705]
                            tunnel: w655 -> [w704]
                            frame #0 {
                              n128 = case shown="0, Default" w657 {
                                tunnel: [w665 w673 w681 w683 w687 w691] -> w658
                                frame 0, Default {
                                n129 = local read "RAM"() -> (w659:bool)
                                n130 = Number To Hexadecimal String(1:i16 4 ("width (-)"), 2:"P (PB1) Sollwert") -> (0:w666:string)
                                n131 = Select(t="*P17", s=w659, f="*W17") -> (s? t:f=w660:string)
                                n132 = Concatenate Strings(w660, w666) -> (w665:string)
                                }
                                frame 1 {
                                n133 = local read "RAM"() -> (w667:bool)
                                n134 = Number To Hexadecimal String(1:i16 4 ("width (-)"), 2:"I ( Reset1) Sollwert") -> (0:w674:string)
                                n135 = Select(t="*P18", s=w667, f="*W18") -> (s? t:f=w669:string)
                                n136 = Concatenate Strings(w669, w674) -> (w673:string)
                                }
                                frame 2 {
                                n137 = local read "RAM"() -> (w676:bool)
                                n138 = Number To Hexadecimal String(1:i16 4 ("width (-)"), 2:"D (Rate) Sollwert") -> (0:w682:string)
                                n139 = Select(t="*P19", s=w676, f="*W19") -> (s? t:f=w677:string)
                                n140 = Concatenate Strings(w677, w682) -> (w681:string)
                                }
                                frame 3 {
                                n141 = local read "RAM"() -> (w686:bool)
                                n142 = Select(t="*G17", s=w686, f="*R17") -> (s? t:f=w683:string)
                                }
                                frame 4 {
                                n143 = local read "RAM"() -> (w690:bool)
                                n144 = Select(t="*G18", s=w690, f="*R18") -> (s? t:f=w687:string)
                                }
                                frame 5 {
                                n145 = local read "RAM"() -> (w694:bool)
                                n146 = Select(t="*G19", s=w694, f="*R19") -> (s? t:f=w691:string)
                                }
                              }
                            }
                            frame #1 {
                              n147 = Unbundle(w698) -> ("VISA resource name out"=w703:refnum<visa-resource-name>, "error out"=w701:errorcluster, "Delay (ms)"=w702:u32, "Write/\nRead"=w700:bool)
                              n148 = call "I3252_Comm_Interface.vi"("VISA resource name in"=w703, "error in"=w701, "Delay (ms)"=w702, "Write"=w700, "String to Write"=w699, "Read"=w700) -> ("VISA resource name out"=w696:refnum<visa-resource-name>, "error out"=w697:errorcluster, "Read String"=w695:string)  [unwired: 2 in]
                            }
                            frame #2 {
                              n149 = case shown="5" w704 {
                                tunnel: w705 -> [_ w709 w713 w717]
                                frame 0, Default {
                                }
                                frame 3 {
                                n150 = String Subset(string=w709, offset (0)=3) -> (substring=w707:string)  [unwired: 1 in]
                                n151 = Hexadecimal String To Number(string=w707) -> (number=→"P (PB1) Istwert":u32)  [unwired: 2 in, 1 out]
                                }
                                frame 4 {
                                n152 = String Subset(string=w713, offset (0)=3) -> (substring=w711:string)  [unwired: 1 in]
                                n153 = Hexadecimal String To Number(string=w711) -> (number=→"I ( Reset1) Istwert":u32)  [unwired: 2 in, 1 out]
                                }
                                frame 5 {
                                n154 = String Subset(string=w717, offset (0)=3) -> (substring=w715:string)  [unwired: 1 in]
                                n155 = Hexadecimal String To Number(string=w715) -> (number=→"D (Rate) IstWert":u32)  [unwired: 2 in, 1 out]
                                }
                              }
                            }
                          }
                        }
                      }
                      frame #2 {
                        n156 = property on="Set PID" class="Bool"("Blinking"=FALSE) -> ()  [unwired: 2 in, 2 out]
                      }
                    }
                    n157 = Not(x="Set PID") -> (.not. x?=w644:bool)
                  }
                  event "Get Values": Value Change {
                    n158 = event-data() -> ()  [unwired: 1 in, 1 out]
                    n159 = stacked-sequence {
                      tunnel: w721 -> [_ w728 _]
                      tunnel: [_ w727 _] -> w720
                      tunnel: [_ w726 _] -> w719
                      frame #0 {
                        n160 = property on="Get Values" class="Bool"("Blinking"=TRUE) -> ()  [unwired: 2 in, 2 out]
                        n161 = property on="ON" class="Bool (strict)"("Blinking"=FALSE) -> ()  [unwired: 2 in, 2 out]
                      }
                      frame #1 {
                        n162 = for {
                          N: 6 -> [_]
                          tunnel: w728 -> [w732]
                          tunnel: [w731] -> w727
                          tunnel: [w730] -> w726
                          i -> [w734]
                          n163 = flat-sequence {
                            tunnel: w734 -> [w736]
                            tunnel: [w737] -> w733
                            tunnel: w733 -> [w759]
                            tunnel: [w760] -> w735
                            tunnel: w732 -> [w758]
                            tunnel: [w757] -> w730
                            tunnel: [w756] -> w731
                            tunnel: w735 -> [w766]
                            tunnel: w734 -> [w765]
                            frame #0 {
                              n164 = case shown="0, Default" w736 {
                                tunnel: [w740 w744 w748 "*R27" "*R28" w754] -> w737
                                frame 0, Default {
                                n165 = local read "RAM"() -> (w741:bool)
                                n166 = Select(t="*G17", s=w741, f="*R17") -> (s? t:f=w740:string)
                                }
                                frame 1 {
                                n167 = local read "RAM"() -> (w745:bool)
                                n168 = Select(t="*G18", s=w745, f="*R18") -> (s? t:f=w744:string)
                                }
                                frame 2 {
                                n169 = local read "RAM"() -> (w749:bool)
                                n170 = Select(t="*G19", s=w749, f="*R19") -> (s? t:f=w748:string)
                                }
                                frame 3 {
                                }
                                frame 4 {
                                }
                                frame 5 {
                                n171 = local read "RAM"() -> (w755:bool)
                                n172 = Select(t="*G01", s=w755, f="*R01") -> (s? t:f=w754:string)
                                }
                              }
                            }
                            frame #1 {
                              n173 = Unbundle(w758) -> ("VISA resource name out"=w764:refnum<visa-resource-name>, "error out"=w762:errorcluster, "Delay (ms)"=w763:u32, "Write/\nRead"=w761:bool)
                              n174 = call "I3252_Comm_Interface.vi"("VISA resource name in"=w764, "error in"=w762, "Delay (ms)"=w763, "Write"=w761, "String to Write"=w759, "Read"=w761) -> ("VISA resource name out"=w756:refnum<visa-resource-name>, "error out"=w757:errorcluster, "Read String"=w760:string)  [unwired: 2 in]
                            }
                            frame #2 {
                              n175 = case shown="0, Default" w765 {
                                tunnel: w766 -> [w768 w772 w776 w780 w784 w788]
                                frame 0, Default {
                                n176 = String Subset(string=w768, offset (0)=3) -> (substring=w769:string)  [unwired: 1 in]
                                n177 = Hexadecimal String To Number(string=w769) -> (number=w767:u32)  [unwired: 2 in, 1 out]
                                n178 = local write "P (PB1) Sollwert"(w767) -> ()
                                n179 = local write "P (PB1) Istwert"(w767) -> ()
                                }
                                frame 1 {
                                n180 = String Subset(string=w772, offset (0)=3) -> (substring=w773:string)  [unwired: 1 in]
                                n181 = Hexadecimal String To Number(string=w773) -> (number=w771:u32)  [unwired: 2 in, 1 out]
                                n182 = local write "I ( Reset1) Sollwert"(w771) -> ()
                                n183 = local write "I ( Reset1) Istwert"(w771) -> ()
                                }
                                frame 2 {
                                n184 = String Subset(string=w776, offset (0)=3) -> (substring=w777:string)  [unwired: 1 in]
                                n185 = Hexadecimal String To Number(string=w777) -> (number=w775:u32)  [unwired: 2 in, 1 out]
                                n186 = local write "D (Rate) Sollwert"(w775) -> ()
                                n187 = local write "D (Rate) IstWert"(w775) -> ()
                                }
                                frame 3 {
                                n188 = String Subset(string=w780, offset (0)=3) -> (substring=w781:string)  [unwired: 1 in]
                                n189 = Hexadecimal String To Number(string=w781) -> (number=w779:u32)  [unwired: 2 in, 1 out]
                                n190 = local write "% LOW Istwert"(w779) -> ()
                                n191 = local write "% LOW Sollwert"(w779) -> ()
                                }
                                frame 4 {
                                n192 = String Subset(string=w784, offset (0)=3) -> (substring=w785:string)  [unwired: 1 in]
                                n193 = Hexadecimal String To Number(string=w785) -> (number=w783:u32)  [unwired: 2 in, 1 out]
                                n194 = local write "% High Sollwert"(w783) -> ()
                                n195 = local write "% HIGH Istwert"(w783) -> ()
                                }
                                frame 5 {
                                n196 = call "I3252_Edit_Setpoint.vi"("Read String"=w788) -> ("Setpoint is"=w787:dbl)
                                n197 = local write "SP 1 is (°C)"(w787) -> ()
                                }
                              }
                            }
                          }
                        }
                      }
                      frame #2 {
                        n198 = property on="Get Values" class="Bool"("Blinking"=FALSE) -> ()  [unwired: 2 in, 2 out]
                      }
                    }
                    n199 = Not(x="Get Values") -> (.not. x?=w723:bool)
                  }
                  event "RAM": Value Change {
                    n200 = event-data() -> ()  [unwired: 1 in, 1 out]
                    n201 = stacked-sequence {
                      tunnel: w792 -> [_ w799 _]
                      tunnel: [_ w798 _] -> w791
                      tunnel: [_ w797 _] -> w790
                      frame #0 {
                        n202 = property on="RAM" class="Bool (strict)"("Blinking"=TRUE) -> ()  [unwired: 2 in, 2 out]
                        n203 = property on="ON" class="Bool (strict)"("Blinking"=FALSE) -> ()  [unwired: 2 in, 2 out]
                      }
                      frame #1 {
                        n204 = for {
                          N: 6 -> [_]
                          tunnel: w799 -> [w803]
                          tunnel: [w802] -> w798
                          tunnel: [w801] -> w797
                          i -> [w805]
                          n205 = flat-sequence {
                            tunnel: w805 -> [w807]
                            tunnel: [w808] -> w804
                            tunnel: w804 -> [w827]
                            tunnel: [w828] -> w806
                            tunnel: w803 -> [w831]
                            tunnel: [w830] -> w801
                            tunnel: [w829] -> w802
                            tunnel: w806 -> [w837]
                            tunnel: w805 -> [w836]
                            frame #0 {
                              n206 = case shown="0, Default" w807 {
                                tunnel: [w811 w815 w819 "*R27" "*R28" w825] -> w808
                                frame 0, Default {
                                n207 = local read "RAM"() -> (w812:bool)
                                n208 = Select(t="*G17", s=w812, f="*R17") -> (s? t:f=w811:string)
                                }
                                frame 1 {
                                n209 = local read "RAM"() -> (w816:bool)
                                n210 = Select(t="*G18", s=w816, f="*R18") -> (s? t:f=w815:string)
                                }
                                frame 2 {
                                n211 = local read "RAM"() -> (w820:bool)
                                n212 = Select(t="*G19", s=w820, f="*R19") -> (s? t:f=w819:string)
                                }
                                frame 3 {
                                }
                                frame 4 {
                                }
                                frame 5 {
                                n213 = local read "RAM"() -> (w826:bool)
                                n214 = Select(t="*G01", s=w826, f="*R01") -> (s? t:f=w825:string)
                                }
                              }
                            }
                            frame #1 {
                              n215 = Unbundle(w831) -> ("VISA resource name out"=w835:refnum<visa-resource-name>, "error out"=w833:errorcluster, "Delay (ms)"=w834:u32, "Write/\nRead"=w832:bool)
                              n216 = call "I3252_Comm_Interface.vi"("VISA resource name in"=w835, "error in"=w833, "Delay (ms)"=w834, "Write"=w832, "String to Write"=w827, "Read"=w832) -> ("VISA resource name out"=w829:refnum<visa-resource-name>, "error out"=w830:errorcluster, "Read String"=w828:string)  [unwired: 2 in]
                            }
                            frame #2 {
                              n217 = case shown="0, Default" w836 {
                                tunnel: w837 -> [w839 w843 w847 w851 w855 w859]
                                frame 0, Default {
                                n218 = String Subset(string=w839, offset (0)=3) -> (substring=w840:string)  [unwired: 1 in]
                                n219 = Hexadecimal String To Number(string=w840) -> (number=w838:u32)  [unwired: 2 in, 1 out]
                                n220 = local write "P (PB1) Sollwert"(w838) -> ()
                                n221 = local write "P (PB1) Istwert"(w838) -> ()
                                }
                                frame 1 {
                                n222 = String Subset(string=w843, offset (0)=3) -> (substring=w844:string)  [unwired: 1 in]
                                n223 = Hexadecimal String To Number(string=w844) -> (number=w842:u32)  [unwired: 2 in, 1 out]
                                n224 = local write "I ( Reset1) Sollwert"(w842) -> ()
                                n225 = local write "I ( Reset1) Istwert"(w842) -> ()
                                }
                                frame 2 {
                                n226 = String Subset(string=w847, offset (0)=3) -> (substring=w848:string)  [unwired: 1 in]
                                n227 = Hexadecimal String To Number(string=w848) -> (number=w846:u32)  [unwired: 2 in, 1 out]
                                n228 = local write "D (Rate) IstWert"(w846) -> ()
                                n229 = local write "D (Rate) Sollwert"(w846) -> ()
                                }
                                frame 3 {
                                n230 = String Subset(string=w851, offset (0)=3) -> (substring=w852:string)  [unwired: 1 in]
                                n231 = Hexadecimal String To Number(string=w852) -> (number=w850:u32)  [unwired: 2 in, 1 out]
                                n232 = local write "% LOW Istwert"(w850) -> ()
                                n233 = local write "% LOW Sollwert"(w850) -> ()
                                }
                                frame 4 {
                                n234 = String Subset(string=w855, offset (0)=3) -> (substring=w856:string)  [unwired: 1 in]
                                n235 = Hexadecimal String To Number(string=w856) -> (number=w854:u32)  [unwired: 2 in, 1 out]
                                n236 = local write "% HIGH Istwert"(w854) -> ()
                                n237 = local write "% High Sollwert"(w854) -> ()
                                }
                                frame 5 {
                                n238 = call "I3252_Edit_Setpoint.vi"("Read String"=w859) -> ("Setpoint is"=w858:dbl)
                                n239 = local write "SP 1 is (°C)"(w858) -> ()
                                }
                              }
                            }
                          }
                        }
                      }
                      frame #2 {
                        n240 = property on="RAM" class="Bool (strict)"("Blinking"=FALSE) -> ()  [unwired: 2 in, 2 out]
                      }
                    }
                    n241 = Not(x="RAM") -> (.not. x?=w794:bool)
                  }
                  event "Set Gauge to Zero": Value Change {
                    n242 = event-data() -> ()  [unwired: 1 in, 1 out]
                    n243 = flat-sequence {
                      tunnel: w865 -> [w870]
                      tunnel: [w870] -> w864
                      tunnel: w864 -> [w872]
                      tunnel: [w876] -> w863
                      tunnel: [w875] -> w862
                      tunnel: [w872] -> w861
                      tunnel: w863 -> [w882]
                      tunnel: w862 -> [w881]
                      tunnel: w861 -> [w877]
                      frame #0 {
                        n244 = property on="Set Gauge to Zero" class="Bool"("Blinking"=TRUE) -> ()  [unwired: 2 in, 2 out]
                      }
                      frame #1 {
                        w873 = 0 items=["sensor 1", "sensor 2", "test"] ("Sensor Nr.:")
                        n245 = call "DUAL GAUGE-Get Pressure,Status.vi"("Sensor Nr.:"=w873, "Referenz in"=w872) -> ("Pressure"=w876:dbl)  [unwired: 6 in, 3 out]
                        n246 = call "DUAL GAUGE-Offset display.vi"("W/R"=FALSE, "Referenz in"=w872) -> ("Sensor 1 Get"=w875:dbl)  [unwired: 6 in, 3 out]
                      }
                      frame #2 {
                        n247 = Add(x=w882, y=w881) -> (x+y=w878:dbl)
                        n248 = call "DUAL GAUGE-Offset display.vi"("W/R"=TRUE, "Sensor 1 Set"=w878, "Referenz in"=w877) -> ("Sensor 1 Get"=→"Current Offset (mbar)":dbl)  [unwired: 5 in, 3 out]
                      }
                      frame #3 {
                        n249 = property on="Set Gauge to Zero" class="Bool"("Blinking"=TRUE) -> ()  [unwired: 2 in, 2 out]
                      }
                    }
                    n250 = Unbundle(w869) -> ("VISA resource name out"=w868:refnum<visa-resource-name>, "error out"=w867:errorcluster)  [unwired: 2 out]
                  }
                  event "Write to File": Value Change {
                    n251 = event-data() -> ("NewVal"=w888:bool)  [unwired: 1 in]
                    n252 = Unbundle(w891) -> ("VISA resource name out"=w890:refnum<visa-resource-name>, "error out"=w889:errorcluster)  [unwired: 2 out]
                    n253 = local read "File Path"() -> (w884:path)
                    n254 = case shown="True" w888 {
                      tunnel: w884 -> [_ w896]
                      tunnel: "User" -> [_ w895]
                      tunnel: "Sample" -> [_ w894]
                      tunnel: [path "" ("File Path") w893] -> w885
                      frame False {
                      }
                      frame True {
                        n255 = call "Header.vi"("Sample"=w894, "User"=w895, "File Path"=w896) -> ("File Path"=w893:path)
                      }
                    }
                    n256 = local write "File Path"(w885) -> ()
                  }
                }
              }
              n257 = Bundle(cluster=w390, "VISA resource name out"=w389, "error out"=w388) -> (w387:T7)  [unwired: 2 in]
            }
            frame #2 {
            }
            frame #3 {
              (unwired) "Daniel Schuster (geb. 20.03.1988)"
              n258 = node-c288(w949) -> (w958:T3)  [unwired: 2 in]
              n259 = node-c288(w964) -> (w967:T3)  [unwired: 2 in]
              n260 = node-c288(w954) -> (w956:T3)  [unwired: 2 in]
              n261 = node-c288(w963) -> (w971:T3)  [unwired: 2 in]
              n262 = timed-sequence {
                timing: w958 -> [_]
                timing-out: [_] -> w957
                tunnel: w933 -> [w1014]
                tunnel: w932 -> [w1010]
                tunnel: [w1013] -> w925
                tunnel: w924 -> [w1012]
                tunnel: w923 -> [w1011]
                tunnel: [w1009] -> w922
                tunnel: [w1008] -> w921
                tunnel: [w1007] -> w919
                n263 = timed-flat-sequence {
                  tunnel: w1014 -> [w1023]
                  tunnel: [w1022] -> w1013
                  tunnel: w1012 -> [w1021]
                  tunnel: w1011 -> [w1020]
                  tunnel: w1010 -> [w1019]
                  tunnel: [w1017] -> w1009
                  tunnel: [w1016] -> w1008
                  tunnel: [w1015] -> w1007
                  n264 = node-c288() -> ()  [unwired: 1 in, 1 out]
                  n265 = case shown="True" "ON (TPG 2)" {
                    tunnel: w1019 -> [w1028 w1034]
                    tunnel: w1020 -> [w1027 w1033]
                    tunnel: [w1026 w1032] -> w1016
                    tunnel: [w1025 w1031] -> w1015
                    frame False {
                      w1029 = 0.0 ("Pressure")
                      n266 = property on="ON (TPG 2)" class="Bool (strict)"("Blinking"=FALSE) -> ()  [unwired: 2 in, 2 out]
                      n267 = Bundle("Pressure"=w1029, "Pressure"=w1029) -> (w1026:cluster{"Pressure":dbl, "Pressure":dbl})  [unwired: 1 in]
                      n268 = Bundle("TPG 2 COM"=w1028, "error out"=w1027) -> (w1025:T9)  [unwired: 1 in]
                    }
                    frame True {
                      n269 = stacked-sequence {
                        tunnel: w1034 -> [_ w1047]
                        tunnel: [_ w1043] -> w1032
                        tunnel: [_ w1039] -> w1031
                        tunnel: w1033 -> [_ w1036]
                        frame #0 {
                          n270 = property on="ON (TPG 2)" class="Bool (strict)"("Blinking"=TRUE) -> ()  [unwired: 2 in, 2 out]
                        }
                        frame #1 {
                          n271 = call "PresureGetSubVI.vi"("COM in"=w1047, "Fehler (Eingang)"=w1036) -> ("Status Gauge#1"=→"Status Gauge 2#1":i32, "Status Gauge#2"=→"Status Gauge 2#2":i32, "COM out"=w1040:refnum<visa-resource-name>, "Pressure Gauge#1"=w1041:dbl, "Pressure Gauge#2"=w1044:dbl, "Cluster (Ausgang)"=w1037:errorcluster)  [unwired: 12 in]
                          "Pressure Gauge 2#1" <- w1041
                          "Pressure Gauge 2#2" <- w1044
                          n272 = Bundle("COM out"=w1040, "Cluster (Ausgang)"=w1037) -> (w1039:T10)  [unwired: 1 in]
                          n273 = Unbundle(w1037) -> ("status"=w1038:bool, "code"=w1042:i32)  [unwired: 1 out]
                          n274 = Bundle("status"=w1038, "code"=w1042) -> ()  [unwired: 1 in, 1 out]
                          n275 = Bundle("Pressure Gauge#1"=w1041, "Pressure Gauge#2"=w1044) -> (w1043:T11)  [unwired: 1 in]
                        }
                      }
                    }
                  }
                  n276 = case shown="True" "ON (TPG 1)" {
                    tunnel: w1023 -> [w1051 w1057]
                    tunnel: [w1050 w1056] -> w1022
                    tunnel: w1021 -> [w1049 w1055]
                    tunnel: [w1048 w1054] -> w1017
                    frame False {
                      w1052 = 0.0 ("Pressure")
                      n277 = property on="ON (TPG 1)" class="Bool (strict)"("Blinking"=FALSE) -> ()  [unwired: 2 in, 2 out]
                      n278 = Bundle("Pressure"=w1052, "Pressure"=w1052) -> (w1048:cluster{"Pressure":dbl, "Pressure":dbl})  [unwired: 1 in]
                      n279 = Bundle("TPG 1 COM"=w1051, "error out"=w1049) -> (w1050:T12)  [unwired: 1 in]
                    }
                    frame True {
                      n280 = stacked-sequence {
                        tunnel: w1057 -> [_ w1070]
                        tunnel: [_ w1063] -> w1056
                        tunnel: w1055 -> [_ w1060]
                        tunnel: [_ w1059] -> w1054
                        frame #0 {
                          n281 = property on="ON (TPG 1)" class="Bool (strict)"("Blinking"=TRUE) -> ()  [unwired: 2 in, 2 out]
                        }
                        frame #1 {
                          n282 = call "PresureGetSubVI.vi"("COM in"=w1070, "Fehler (Eingang)"=w1060) -> ("Status Gauge#1"=→"Status Gauge 1#1":i32, "Status Gauge#2"=→"Status Gauge 1#2":i32, "COM out"=w1064:refnum<visa-resource-name>, "Pressure Gauge#1"=w1065:dbl, "Pressure Gauge#2"=w1067:dbl, "Cluster (Ausgang)"=w1061:errorcluster)  [unwired: 12 in]
                          "Pressure Gauge 1#1" <- w1065
                          "Pressure Gauge 1#2" <- w1067
                          n283 = Bundle("COM out"=w1064, "Cluster (Ausgang)"=w1061) -> (w1063:T10)  [unwired: 1 in]
                          n284 = Unbundle(w1061) -> ("status"=w1062:bool, "code"=w1066:i32)  [unwired: 1 out]
                          n285 = Bundle("status"=w1062, "code"=w1066) -> ()  [unwired: 1 in, 1 out]
                          n286 = Bundle("Pressure Gauge#1"=w1065, "Pressure Gauge#2"=w1067) -> (w1059:T11)  [unwired: 1 in]
                        }
                      }
                    }
                  }
                  n287 = node-c288() -> ()  [unwired: 1 in, 1 out]
                }
              }
              n288 = timed-sequence {
                timing: w967 -> [_]
                timing-out: [_] -> w966
                tunnel: w965 -> [w1080]
                tunnel: [w1079] -> w960
                tunnel: [w1078] -> w959
                tunnel: [w1077] -> w946
                n289 = timed-flat-sequence {
                  tunnel: w1080 -> [w1084]
                  tunnel: [w1083] -> w1079
                  tunnel: [w1082] -> w1078
                  tunnel: [w1081] -> w1077
                  n290 = node-c288() -> ()  [unwired: 1 in, 1 out]
                  n291 = case shown="True" "ON" {
                    tunnel: w1084 -> [w1088 w1093]
                    tunnel: [w1087 w1092] -> w1083
                    tunnel: [w1086 w1091] -> w1082
                    tunnel: [_ w1090] -> w1081
                    frame False {
                      n292 = Unbundle(w1088) -> ("VISA resource name out"=w1087:refnum<visa-resource-name>, "error out"=w1086:errorcluster)  [unwired: 2 out]
                      n293 = property on="ON" class="Bool (strict)"("Blinking"=FALSE) -> ()  [unwired: 2 in, 2 out]
                    }
                    frame True {
                      n294 = stacked-sequence {
                        tunnel: w1093 -> [_ w1098]
                        tunnel: [_ w1097] -> w1092
                        tunnel: [_ w1096] -> w1091
                        tunnel: [_ w1095] -> w1090
                        frame #0 {
                          n295 = property on="ON" class="Bool (strict)"("Blinking"=TRUE) -> ()  [unwired: 2 in, 2 out]
                        }
                        frame #1 {
                          n296 = Unbundle(w1098) -> ("VISA resource name out"=w1102:refnum<visa-resource-name>, "error out"=w1100:errorcluster, "Delay (ms)"=w1101:u32, "Write/\nRead"=w1099:bool)
                          n297 = call "I3252_Comm_Interface.vi"("VISA resource name in"=w1102, "error in"=w1100, "Delay (ms)"=w1101, "Write"=w1099, "String to Write"="*V01", "Read"=w1099) -> ("VISA resource name out"=w1097:refnum<visa-resource-name>, "error out"=w1096:errorcluster, "Read String"=w1095:string)  [unwired: 2 in]
                        }
                      }
                    }
                  }
                  n298 = node-c288() -> ()  [unwired: 1 in, 1 out]
                }
              }
              n299 = timed-sequence {
                timing: w956 -> [_]
                timing-out: [_] -> w955
                tunnel: w953 -> [w976]
                tunnel: w952 -> [w975]
                tunnel: [w974] -> w950
                tunnel: [w973] -> w951
                tunnel: [w972] -> w947
                n300 = timed-flat-sequence {
                  tunnel: w976 -> [w981]
                  tunnel: w975 -> [w980]
                  tunnel: [w979] -> w974
                  tunnel: [w978] -> w973
                  tunnel: [w977] -> w972
                  n301 = node-c288() -> ()  [unwired: 1 in, 1 out]
                  n302 = case shown="False" "ON" {
                    tunnel: w981 -> [w985 w991]
                    tunnel: w980 -> [w986 w990]
                    tunnel: [w985 w989] -> w979
                    tunnel: [w986 w988] -> w978
                    tunnel: [0.0 ("Reading") w987] -> w977
                    frame False {
                      n303 = property on="ON" class="Bool (strict)"("Blinking"=FALSE) -> ()  [unwired: 2 in, 2 out]
                    }
                    frame True {
                      n304 = stacked-sequence {
                        tunnel: w991 -> [_ w998]
                        tunnel: w990 -> [_ w997]
                        tunnel: [_ w996] -> w989
                        tunnel: [_ w995] -> w988
                        tunnel: [_ w993] -> w987
                        frame #0 {
                          n305 = property on="ON" class="Bool (strict)"("Blinking"=TRUE) -> ()  [unwired: 2 in, 2 out]
                        }
                        frame #1 {
                          n306 = call "VC840_Read.vi"("error in (no error)"=w997, "VISA resource name"=w998) -> ("error out"=w995:errorcluster, "Unit"=→"Unit 2":string, "Reading"=w993:dbl, "VISA resource name out"=w996:refnum<visa-resource-name>, "Status"=→"Status 2":T2, "Mode"=→"Mode 2":enum16{"?", "Diode", "Beep", "DC", "AC"})  [unwired: 4 out]
                          "Reading 2" <- w993
                        }
                      }
                    }
                  }
                  n307 = node-c288() -> ()  [unwired: 1 in, 1 out]
                }
              }
              n308 = timed-sequence {
                timing: w971 -> [_]
                timing-out: [_] -> w970
                tunnel: w969 -> [w1114]
                tunnel: w968 -> [w1113]
                tunnel: [w1112] -> w962
                tunnel: [w1111] -> w961
                tunnel: [w1110] -> w948
                n309 = timed-flat-sequence {
                  tunnel: w1114 -> [w1119]
                  tunnel: w1113 -> [w1118]
                  tunnel: [w1117] -> w1112
                  tunnel: [w1116] -> w1111
                  tunnel: [w1115] -> w1110
                  n310 = node-c288() -> ()  [unwired: 1 in, 1 out]
                  n311 = case shown="True" "ON" {
                    tunnel: w1119 -> [w1123 w1129]
                    tunnel: w1118 -> [w1124 w1128]
                    tunnel: [w1123 w1127] -> w1117
                    tunnel: [w1124 w1126] -> w1116
                    tunnel: [0.0 ("Reading") w1125] -> w1115
                    frame False {
                      n312 = property on="ON" class="Bool (strict)"("Blinking"=FALSE) -> ()  [unwired: 2 in, 2 out]
                    }
                    frame True {
                      n313 = stacked-sequence {
                        tunnel: w1129 -> [_ w1136]
                        tunnel: w1128 -> [_ w1135]
                        tunnel: [_ w1134] -> w1127
                        tunnel: [_ w1133] -> w1126
                        tunnel: [_ w1131] -> w1125
                        frame #0 {
                          n314 = property on="ON" class="Bool (strict)"("Blinking"=TRUE) -> ()  [unwired: 2 in, 2 out]
                        }
                        frame #1 {
                          n315 = call "VC840_Read.vi"("error in (no error)"=w1135, "VISA resource name"=w1136) -> ("error out"=w1133:errorcluster, "Unit"=→"Unit 1":string, "Reading"=w1131:dbl, "VISA resource name out"=w1134:refnum<visa-resource-name>, "Status"=→"Status 1":T2, "Mode"=→"Mode 1":enum16{"?", "Diode", "Beep", "DC", "AC"})  [unwired: 4 out]
                          "Reading 1" <- w1131
                        }
                      }
                    }
                  }
                  n316 = node-c288() -> ()  [unwired: 1 in, 1 out]
                }
              }
              n317 = Tick Count (ms)() -> (millisecond timer value=w934:u32)
              n318 = Subtract(x=w934, y=w939) -> (x-y=w938:u32)
              n319 = Divide(x=w938, y=u32 1000) -> (x/y=w936:dbl)
              n320 = node-c288(w970) -> ()  [unwired: 1 out]
              n321 = node-c288(w955) -> ()  [unwired: 1 out]
              n322 = node-c288(w966) -> ()  [unwired: 1 out]
              n323 = To Double Precision Float(number=w936) -> (double precision float=w940:dbl)
              "current time (s)" <- w940
              n324 = node-c288(w957) -> ()  [unwired: 1 out]
              n325 = Unbundle(w921) -> ("Pressure Gauge#1"=w920:dbl, "Pressure Gauge#2"=w918:dbl)
              "Pressure OpenPort2" <- w918
              "Pressure Pirani 2" <- w920
              n326 = Unbundle(w922) -> ("Pressure Gauge#1"=w931:dbl, "Pressure Gauge#2"=w926:dbl)
              "Pressure Baratron 2" <- w931
              "Pressure FullRange 2" <- w926
            }
            frame #4 {
              n327 = Build Array (concatenate)(w1156, w1160) -> (w1155:dbl[])
              n328 = Build Array (concatenate)(w1159, w1161) -> (w1154:dbl[])
              n329 = Build Array (concatenate)(w1157, w1148) -> (w1152:dbl[])
              n330 = Build Array (concatenate)(w1158, w1149) -> (w1153:dbl[])
              n331 = Greater?(x=w1180, y="Pressure Limit (mbar)") -> (0:w1183:bool)
              n332 = case shown="False" w1183 {
                frame False {
                  n333 = property on="Standby" class="Bool (strict)"("DisabledEnum"=T6."Enabled" ("Disabled")) -> ()  [unwired: 2 in, 2 out]
                }
                frame True {
                  n334 = property on="Standby" class="Bool (strict)"("Val(Sgnl)"=TRUE ("Standby"), "DisabledEnum"=T6."Disabled" ("Disabled")) -> ()  [unwired: 2 in, 2 out]
                }
              }
              n335 = call "Resistivity_Calculation.vi"("Reading 1 (V)"=w1173, "Constant"="4PP constant", "Thickness (nm)"="Thickness (nm)", "Reading 2 (A)"=w1181) -> ("Resivtivity (Ohm*cm)"=w1165:dbl, "Current"=w1166:dbl, "Voltage"=w1167:dbl)
              "Resistivity (Ohm*cm)" <- w1165
              "Voltage (V)" <- w1167
              "Current (A)" <- w1166
              n336 = call "I3252_Edit_Temperature.vi"("Temp. String"=w1182) -> ("Temp. (°C)"=w1176:dbl)
              "(°C)" <- w1176
              n337 = Build Array (concatenate)(w1178, w1179) -> (w1175:dbl[])
              n338 = Build Array (concatenate)(w1177, w1176) -> (w1163:dbl[])
              n339 = Build Array (concatenate)(w1174, w1167) -> (w1172:dbl[])
              n340 = Build Array (concatenate)(w1171, w1166) -> (w1169:dbl[])
              n341 = Build Array (concatenate)(w1170, w1165) -> (w1168:dbl[])
              n342 = Build Array(w1167, w1166, w1165) -> (w1164:dbl[])
            }
            frame #5 {
              n343 = Bundle(w1211, w1210) -> (→"CMR275 Baratron":cluster{dbl[], dbl[]})  [unwired: 1 in]
              n344 = Bundle(w1211, w1209) -> (→"PKR251 FullRange":cluster{dbl[], dbl[]})  [unwired: 1 in]
              n345 = Bundle(w1211, w1208) -> (→"Pirani (VVP1 Scroll)":cluster{dbl[], dbl[]})  [unwired: 1 in]
              n346 = Bundle(w1211, w1207) -> (→"Pressure OpenPort":cluster{dbl[], dbl[]})  [unwired: 1 in]
              n347 = Bundle(w1211, w1217) -> (→"Thermocouple (Sample holder 1)":cluster{dbl[], dbl[]})  [unwired: 1 in]
              n348 = Bundle(w1211, w1219) -> (→"Voltage":cluster{dbl[], dbl[]})  [unwired: 1 in]
              n349 = Bundle(w1211, w1220) -> (→"Current":cluster{dbl[], dbl[]})  [unwired: 1 in]
              n350 = Bundle(w1211, w1221) -> (→"Resistivity":cluster{dbl[], dbl[]})  [unwired: 1 in]
              n351 = Build Array (concatenate)(w1216, w1226, w1225, w1215, w1202, w1198, w1196) -> (w1233:dbl[])
              "appended array" <- w1233
            }
            frame #6 {
              n352 = Unbundle(w1239) -> ("COM out"=w1238:refnum<visa-resource-name>, "Cluster (Ausgang)"=w1237:errorcluster)
              n353 = Unbundle(w1236) -> ("COM out"=w1235:refnum<visa-resource-name>, "Cluster (Ausgang)"=w1234:errorcluster)
              n354 = case shown="True" "Write to File" {
                tunnel: [_ w1267] -> w1253
                tunnel: "File Path" -> [_ w1265]
                tunnel: w1246 -> [_ w1263]
                frame False {
                  n355 = property on="Write to File" class="Bool (strict)"("Blinking"=FALSE) -> ()  [unwired: 2 in, 2 out]
                }
                frame True {
                  n356 = flat-sequence {
                    tunnel: [w1269] -> w1266
                    tunnel: w1265 -> [w1269]
                    tunnel: [w1268] -> w1264
                    tunnel: w1263 -> [w1268]
                    tunnel: [w1274] -> w1267
                    tunnel: w1266 -> [w1273]
                    tunnel: w1264 -> [w1272]
                    frame #0 {
                      n357 = property on="Write to File" class="Bool (strict)"("Blinking"=TRUE) -> ()  [unwired: 2 in, 2 out]
                    }
                    frame #1 {
                      n358 = call-poly <vilib>:"Write To Spreadsheet File.vi"("format (%.3f)"="%g", "append to file? (new file:F)"=TRUE ("transpose? (no:F)"), "1D data"=w1272, "file path (dialog if empty)"=w1273) -> ("new file path (Not A Path if cancelled)"=w1274:path)  [unwired: 4 in]
                    }
                  }
                }
              }
              n359 = Merge Errors(w1258, w1257, w1255, w1237, w1234) -> (w1256:errorcluster)
              n360 = call <vilib>:"Simple Error Handler.vi"("error in (no error)"=w1256) -> ("error?"=w1240:bool)  [unwired: 4 in, 4 out]
              n361 = local write "File Path"(w1253) -> ()
            }
            frame #7 {
              w1290 = u32 1000 ("y")
              n362 = Tick Count (ms)() -> (millisecond timer value=w1292:u32)
              n363 = Subtract(x=w1292, y=w1291) -> (x-y=w1293:u32)
              n364 = VISA Flush I/O Buffer(VISA resource name=w1284, error in (no error)=w1283) -> (VISA resource name out=w1281:refnum<visa-resource-name>, error out=w1282:errorcluster)  [unwired: 1 in]
              n365 = VISA Flush I/O Buffer(VISA resource name=w1277, error in (no error)=w1276) -> (VISA resource name out=w1280:refnum<visa-resource-name>, error out=w1279:errorcluster)  [unwired: 1 in]
              n366 = Divide(x=w1293, y=w1290) -> (x/y=→"loop time (s)":dbl)
              n367 = Subtract(x="Intervall (s)", y=u32 1) -> (x-y=w1294:u32)
              n368 = Multiply(x=w1294, y=w1290) -> (x*y=w1297:u32)
              n369 = Wait (ms)(milliseconds to wait=w1297) -> ()  [unwired: 1 out]
              n370 = Bundle("COM out"=w1281, "error out"=w1282, "COM out"=w1280, "error out"=w1279) -> (w1278:T13)  [unwired: 1 in]
            }
            frame #8 {
              n371 = Tick Count (ms)() -> (millisecond timer value=w1317:u32)
              n372 = Subtract(x=w1317, y=w1315) -> (x-y=w1316:u32)
              n373 = Divide(x=w1316, y=w1314) -> (x/y=→"data logger intervall (s)":dbl)
            }
          }
          n374 = Exclusive Or(1:"stop", 2:w153) -> (0:w154:bool)
        }
      }
      frame #4 {
        n375 = call "VC840_Close.vi"("error in (no error)"=w1336, "VISA resource name"=w1337) -> ("error out"=w1345:errorcluster)  [unwired: 9 in]
        n376 = call "VC840_Close.vi"("error in (no error)"=w1338, "VISA resource name"=w1339) -> ("error out"=w1343:errorcluster)  [unwired: 9 in]
        n377 = VISA Close(VISA resource name=w1341, error in (no error)=w1340) -> (error out=w1342:errorcluster)
        n378 = Unbundle(w1334) -> ("COM out"=w1333:refnum<visa-resource-name>, "error out"=w1332:errorcluster, "COM out"=w1330:refnum<visa-resource-name>, "error out"=w1331:errorcluster)
        n379 = VISA Close(VISA resource name=w1333, error in (no error)=w1332) -> ()  [unwired: 1 out]
        n380 = VISA Close(VISA resource name=w1330, error in (no error)=w1331) -> ()  [unwired: 1 out]
        n381 = Merge Errors(w1342, w1343, w1345) -> (w1344:errorcluster)
        n382 = call <vilib>:"Simple Error Handler.vi"("error in (no error)"=w1344) -> ("error?"=w1335:bool)  [unwired: 1 in, 7 out]
        n383 = Stop(stop? (T)=w1335) -> ()
      }
    }
  }
